vi "VFP.vi"() -> ()   [LabVIEW 2009]
uses:
  states/InitializationStates.ctl
  Instance           6 11Saved   VFP .vi
  Instance          21 11Saved   VFP .vi
  Instance           8 11Saved   VFP .vi
  <vilib>/Utility/error.llb/DialogType.ctl
  states/DataAcqStates.ctl
  Instance           5 11Saved   VFP .vi
  <vilib>/registry/registry.llb/Registry SAM.ctl
  <vilib>/registry/registry.llb/Registry RtKey.ctl
  <vilib>/registry/registry.llb/Read Registry Value Simple STR.vi
  Instance          20 11Saved   VFP .vi
  <vilib>/Utility/error.llb/whitespace.ctl
  <vilib>/Analysis/NI_AALPro.lvlib
panel:
  out "Control Amp Overload":bool caption="CA"
  out "Current Overload":bool caption="I"
  out "Voltage Overload":bool caption="V"
  in  "Select Graph":u16(ring) items=["V Vs. T, I vs. T", "I vs. V", "V vs. I"]
  in  "Log Data To File":bool
  out "Family":string
  out "Vf History":sgl[](array[numeric])
  out "Im History":sgl[](array[numeric])
  out "XY Graph Flipped?":bool
  in  "CA Speed":u16(ring)
  in  "I/E Stability":u16(ring)=2 items=["Fast", "Medium Fast", "Normal", "Slow"]
  in  "IchOffsetEnable":bool
  in  "VchOffsetEnable":bool
  in  "Ich Offset":sgl step=0.1 format="%^.3e"
  in  "Vch Offset":sgl step=0.1 format="%^.3e"
  in  "Ich Filter":u16(ring)
  in  "Vch Filter":u16(ring)
  in  "Ich Autorange":bool
  in  "Vch Autorange":bool
  in  "I/E Autorange":bool
  in  "I/E Range":u16(ring)
  in  "Ich Range":u16(ring)
  in  "Vch Range":u16(ring)
  in  "Device":u16(ring)
  in  "CtrlMode":u32(ring)=1 items=["Galvanostat", "Potentiostat", "ZRA"]
  in  "Continuous":bool=TRUE
  in  "Acq. Frequency":dbl=100.0 caption="Hz" min=0.001667 max=10000.0 step=1.0 format="%.3f"
  in  "Cycles":u32=1 min=1 step=1
  in  "Signal Type":u16(ring) items=["Sine Wave"=0, "Cosine Wave"=1, "Triangle"=2, "Square Wave"=3, "Sawtooth"=4, "Ramp"=5, "Single Point"=7, "From File"=8]
  in  "Filename":path
  in  "Phase Offset":dbl caption="Degrees" step=1.0 format="%.3f"
  in  "DC Offset":dbl caption="V" step=0.1 format="%^.3e"
  in  "Amplitude":dbl=0.1 caption="V" step=0.1 format="%^.3e"
  in  "Signal Frequency":dbl=1.0 caption="Hz" min=5e-05 max=300000.0 step=0.5 format="%.3f"
  in  "Final":dbl=1.0 caption="V" step=0.1 format="%^.3e"
  in  "Initial":dbl caption="V" step=0.1 format="%^.3e"
  in  "Duty Cycle":dbl=50.0 caption="Percent" min=0.0 max=100.0 step=0.1 format="%.3f"
  in  "Scan Rate":dbl=1.0 caption="V/s" step=0.01 format="%_3f"
  in  "Cell State":bool
  in  "Auto Cell Switch":bool=TRUE
  in  "Start/Stop":bool caption="Start"
  out "Confirm Exit?":bool
  out "Vs. T":sgl[][](graph)
  out "I vs. V":cluster{dbl, dbl}[](graph)
  out "SetCell":bool
  out "Cell Val Change NewVal":bool
  out "Version":string
  in  "[user-defined codes]":u32[](array[numeric])=[3758096430]
  in  "[user-defined descriptions]":string[](array[string])=["Device Not Authorized"]
  out "Taking Data":bool
  out "Front Panel Window:Title":string="Gamry Instruments Virtual Front Panel"
  in  "Log File":path
  out "Device Gone":bool
  out "Index of Device (Device Change)":i32
  out "milliseconds to wait":u32=150
  in  "Close":bool
  out "From File Refnum":refnum<file>
  out "Data Handlers":T1
  out "Log File Refnum":refnum<file>
  out "ForcePstatFunctionUpdate":bool
  out "File Data":string
  out "Device List Change Callback":refnum<k27>
  in  "Device List Change":bool
  out "Device Open":bool
  out "Section":string
  in  "GAMRYCOMLib.IGamrySignalArray":refnum<k7>
  in  "GAMRYCOMLib.IGamryDtaqIv":refnum<k7>
  in  "GAMRYCOMLib.IGamryPstat":refnum<k7>
  in  "GAMRYCOMLib.IGamryDeviceList":refnum<k7>
  out "DataDone Callback":refnum<k27>
  out "DataDone?":bool
  out "Dtaq Graph Callback":refnum<k27>
  in  "GAMRYCOMLib.IGamrySignal":refnum<k7>
  out "Signal":refnum<k7>
  out "Dtaq":refnum<k7>
  out "Pstat":refnum<k7>
  out "Device List":refnum<k7>
  out "First I/E Range":i32
  out "Section List":string[](array[string])=["PC5600-00002"]
  # "Overloads"
  # "Data Acquisition"
  # "Signal Generation"
  # "Device Settings"
  # "Experiment Control"
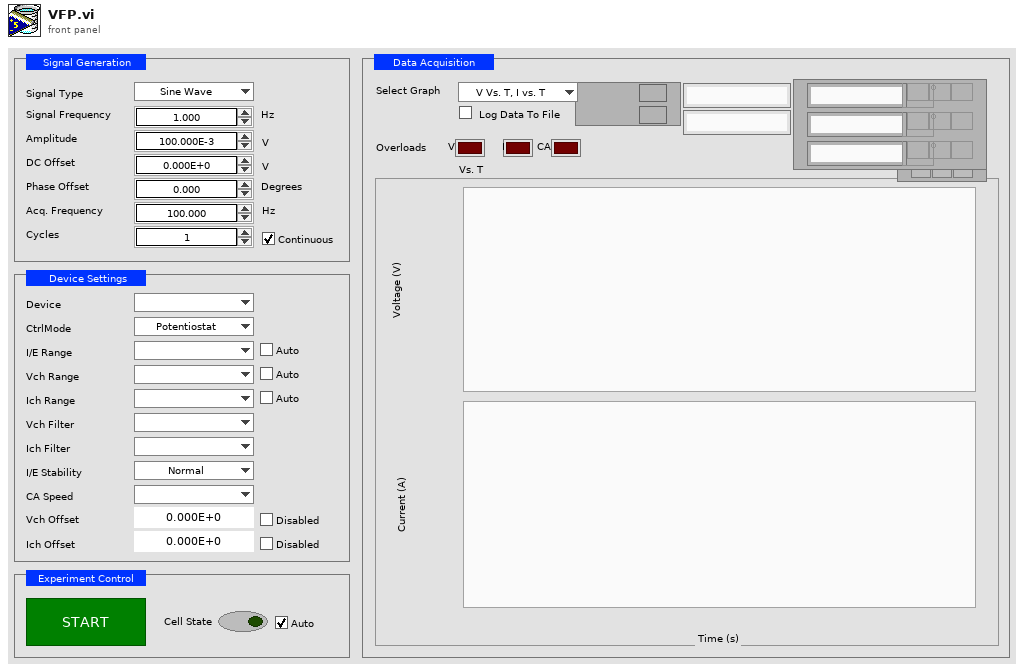
[diagram p1: front panel]
types:
  T1 = cluster{"Vs. T":refnum<vi>, "I vs. V":refnum<vi>, "Log File Refnum":refnum<vi>}
  T2 = typedef "InitializationStates.ctl" = enum16{"Initialize COM", "Load Device List", "Load Range Strings", "Setup Ranges", "Adjust Menu", "STOP"}
  T3 = typedef "DataAcqStates.ctl" = enum16{"Initialize", "Initialize Objects", "Generate Signal", "Data Acq Setup", "Acquire Data", "Cleanup", "STOP"}
  T4 = typedef "Registry SAM.ctl" = enum32{"KEY_QUERY_VALUE", "KEY_SET_VALUE", "KEY_CREATE_SUB_KEY", "KEY_ENUMERATE_SUB_KEYS", "KEY_NOTIFY", "KEY_CREATE_LINK", "KEY_READ", "KEY_WRITE", "KEY_ALL_ACCESS", "KEY_READ | KEY_WRITE"}
  T5 = typedef "Registry RtKey.ctl" = enum32{"HKEY_CLASSES_ROOT", "HKEY_CURRENT_USER", "HKEY_LOCAL_MACHINE", "HKEY_USERS", "HKEY_PERFORMANCE_DATA", "HKEY_CURRENT_CONFIG", "HKEY_DYN_DATA"}
  T6 = enum16{"open", "open or create", "create or replace", "create", "open (read only)"}
  T7 = cluster{"I/E Ranges":string[], "First I/E Range":i32, "VchRanges":string[], "IchRanges":string[], "AchRanges":string[], "VchFilters":string[], "IchFilters":string[], "AchFilters":string[], "Family":string, "CA Speeds":string[]}
  T8 = enum32{"existing file", "new file", "new or existing file", "existing dir", "new dir", "new or existing dir", "existing file (use LLBs)", "new file (use LLBs)", "new or existing file (use LLBs)", "new or existing file or directory (use LLBs)"}
  T9 = typedef "Registry refnum.ctl" = refnum<k1>
  T10 = typedef "whitespace.ctl" = u16
  T11 = cluster{"I Overload":bool, "CA Overload":bool, "V Overload":bool, "I ADC Railed":bool, "V ADC Railed":bool}
  T12 = enum32{"invalid app kind", "Development System", "Run Time System", "Student Edition", "Embedded LabVIEW", "Evaluation", "Custom"}
  T13 = typedef "DialogType.ctl" = u16
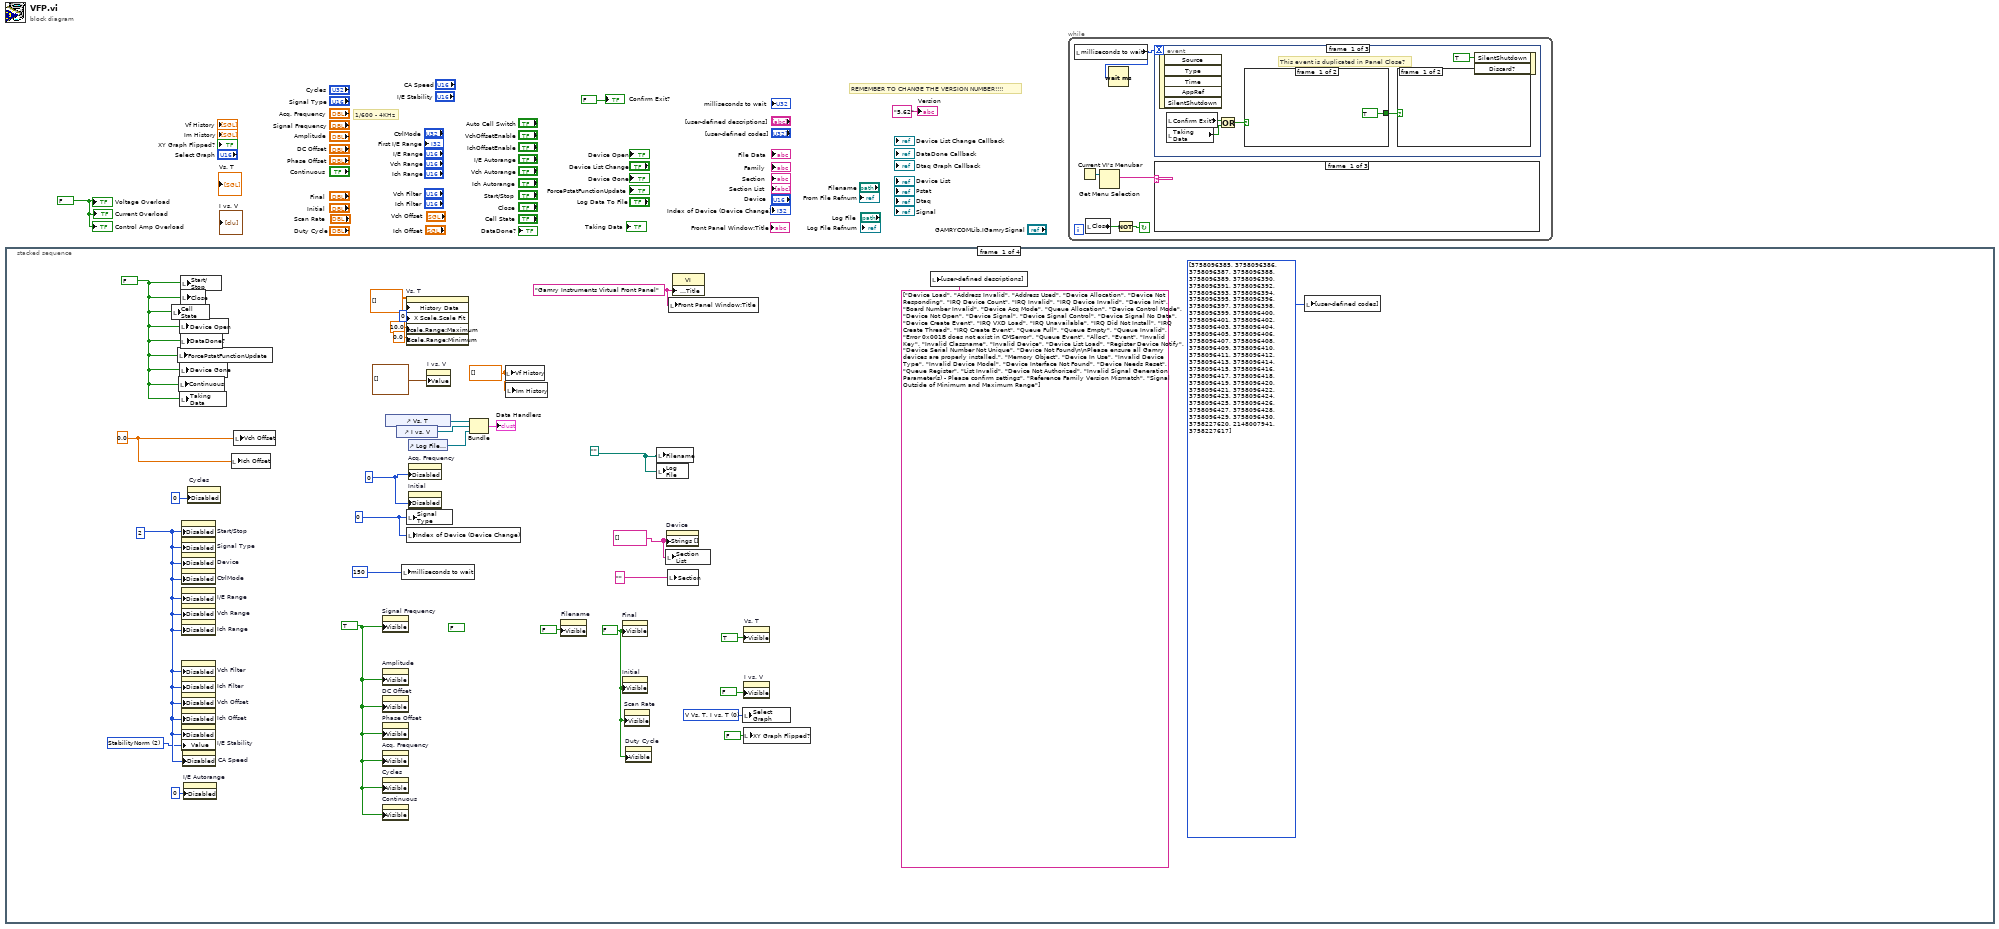
[diagram p0: block diagram]
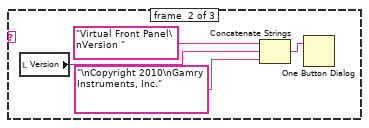
[diagram p2: hidden frame]
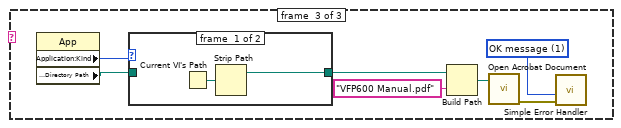
[diagram p3: hidden frame]
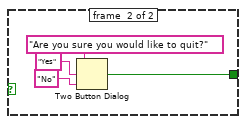
[diagram p5: hidden frame]
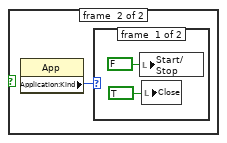
[diagram p6: hidden frame]
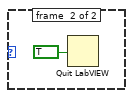
[diagram p7: hidden frame]
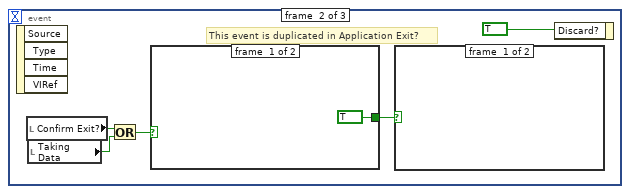
[diagram p8: hidden frame]
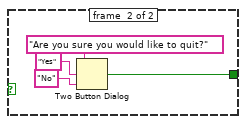
[diagram p9: hidden frame]
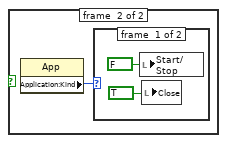
[diagram p10: hidden frame]
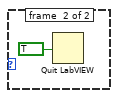
[diagram p11: hidden frame]
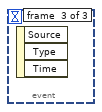
[diagram p12: hidden frame]
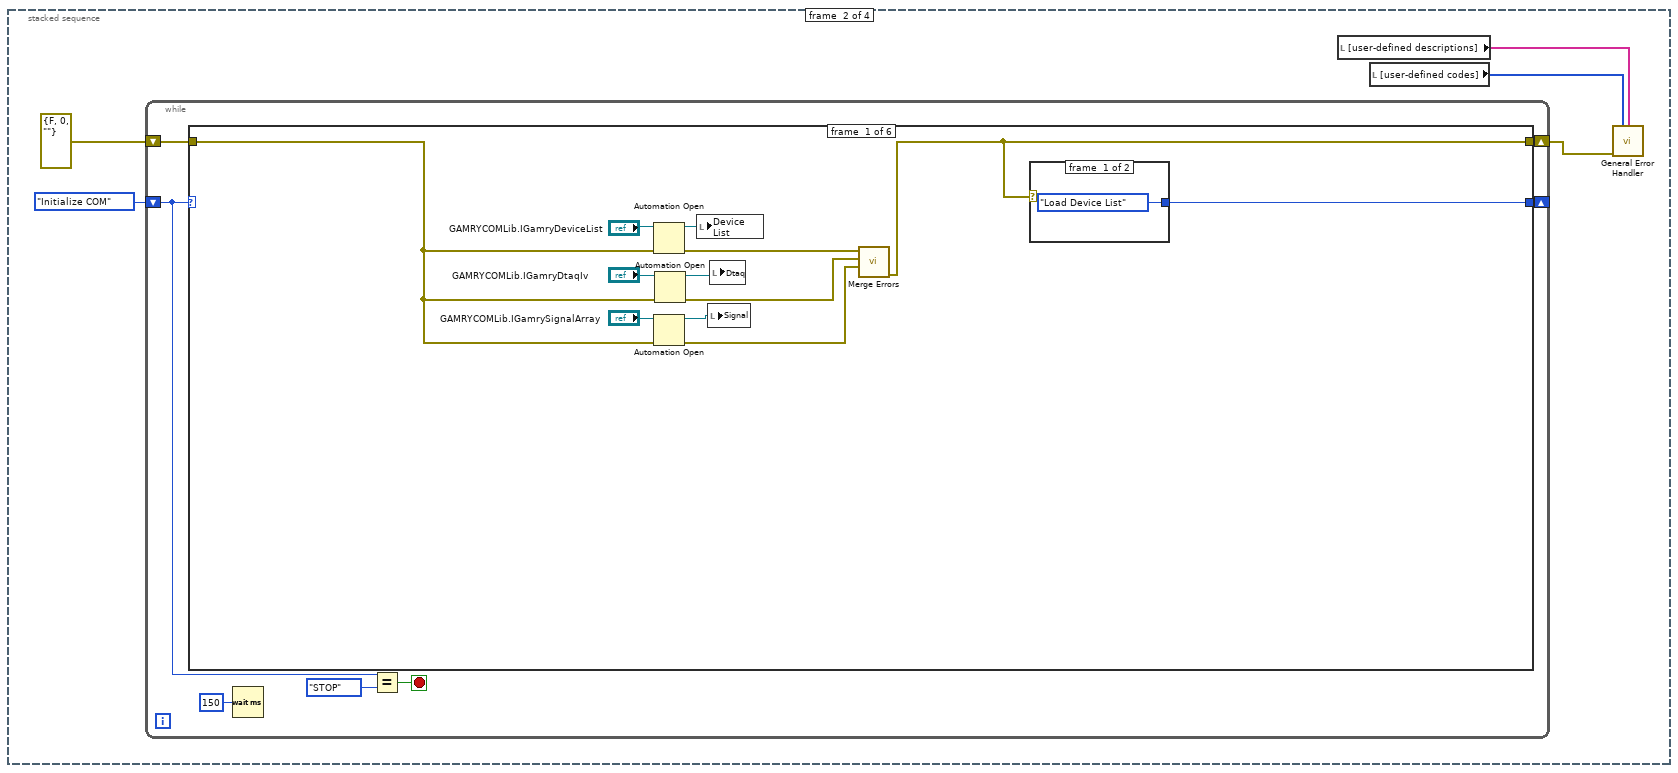
[diagram p13: hidden frame]
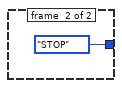
[diagram p14: hidden frame]
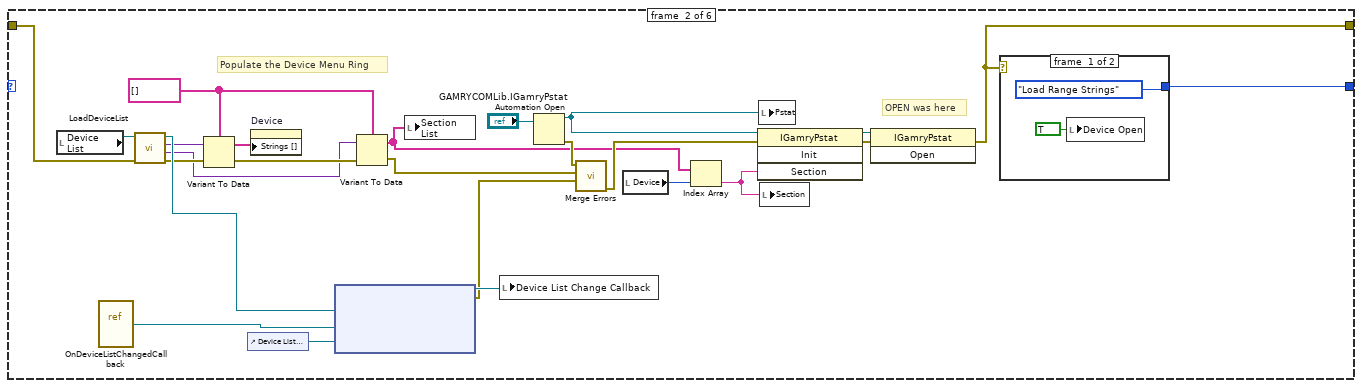
[diagram p15: hidden frame]
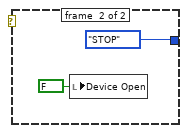
[diagram p16: hidden frame]
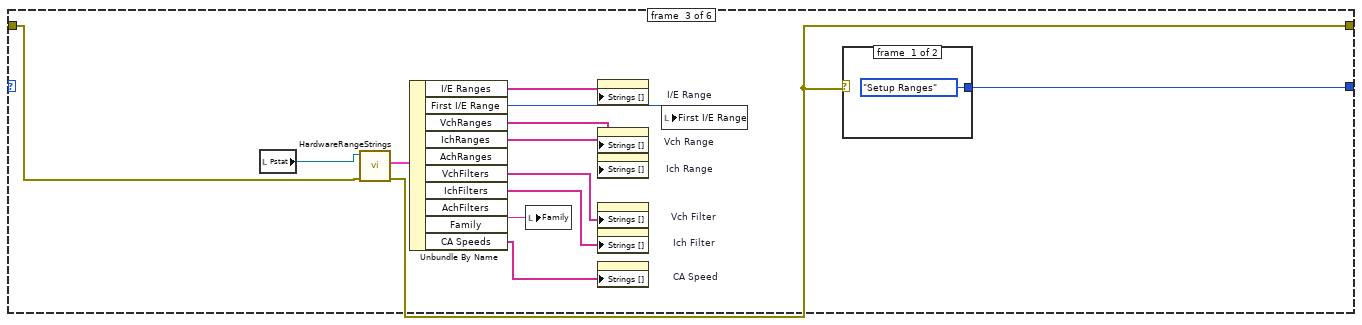
[diagram p17: hidden frame]
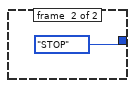
[diagram p18: hidden frame]
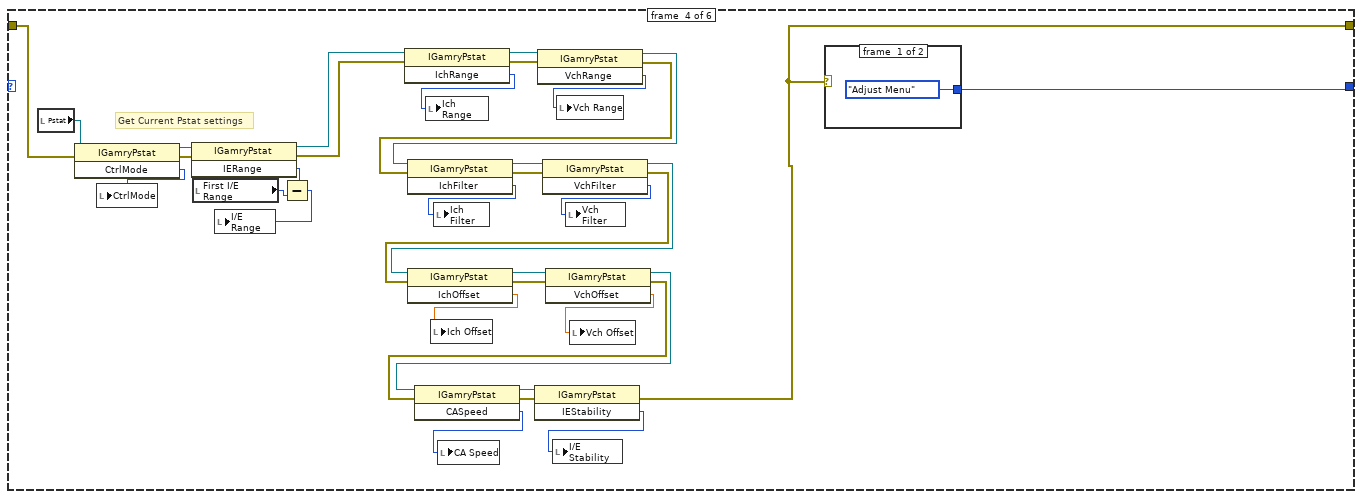
[diagram p19: hidden frame]
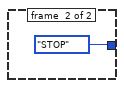
[diagram p20: hidden frame]
diagram:
  w1 = FALSE
  # "REMEMBER TO CHANGE THE VERSION NUMBER!!!!"
  # "1/600 - 4KHz"
  n1 = stacked-sequence {
    frame #0 {
      w5 = sgl[] [] ("Vf History")
      w7 = u16 0 items=["V Vs. T, I vs. T", "I vs. V", "V vs. I"] ("Select Graph")
      w12 = path ""
      w13 = 2 items=["StabilityFast", "StabilityMedFast", "StabilityNorm", "StabilitySlow"] ("Stability")
      w20 = "Gamry Instruments Virtual Front Panel" ("Front Panel Window:Title")
      w15 = FALSE ("Visible")
      w8 = u8 0 ("Disabled")
      w14 = u8 2 ("Disabled")
      (unwired) FALSE ("Visible")
      w30 = TRUE ("Visible")
      w34 = sgl 0.0 ("Vch Offset")
      w19 = FALSE ("I/E Autorange 2")
      w24 = u32 0 ("Zero")
      w25 = string[] [] ("Strings []")
      n2 = local write "Cell State"(w19) -> ()
      n3 = local write "ForcePstatFunctionUpdate"(w19) -> ()
      n4 = local write "Continuous"(w19) -> ()
      n5 = local write "Device Open"(w19) -> ()
      n6 = local write "Device Gone"(w19) -> ()
      n7 = local write "Taking Data"(w19) -> ()
      n8 = local write "DataDone?"(w19) -> ()
      n9 = local write "Start/Stop"(w19) -> ()
      n10 = local write "Close"(w19) -> ()
      n11 = property on="Start/Stop" class="Bool (strict)"("Disabled"=w14) -> ()  [unwired: 2 in, 2 out]
      n12 = property on="Signal Type" class="Ring (strict)"("Disabled"=w14) -> ()  [unwired: 2 in, 2 out]
      n13 = property on="Device" class="Ring (strict)"("Disabled"=w14) -> ()  [unwired: 2 in, 2 out]
      n14 = property on="CtrlMode" class="Ring (strict)"("Disabled"=w14) -> ()  [unwired: 2 in, 2 out]
      n15 = property on="I/E Range" class="Ring (strict)"("Disabled"=w14) -> ()  [unwired: 2 in, 2 out]
      n16 = property on="Vch Range" class="Ring (strict)"("Disabled"=w14) -> ()  [unwired: 2 in, 2 out]
      n17 = property on="Ich Range" class="Ring (strict)"("Disabled"=w14) -> ()  [unwired: 2 in, 2 out]
      n18 = property on="Vch Filter" class="Ring (strict)"("Disabled"=w14) -> ()  [unwired: 2 in, 2 out]
      n19 = property on="Ich Filter" class="Ring (strict)"("Disabled"=w14) -> ()  [unwired: 2 in, 2 out]
      n20 = property on="Vch Offset" class="DigNum (strict)"("Disabled"=w14) -> ()  [unwired: 2 in, 2 out]
      n21 = property on="Ich Offset" class="DigNum (strict)"("Disabled"=w14) -> ()  [unwired: 2 in, 2 out]
      n22 = property on="I/E Stability" class="Ring (strict)"("Disabled"=w14, "Value"=w13) -> ()  [unwired: 2 in, 2 out]
      n23 = property on="CA Speed" class="Ring (strict)"("Disabled"=w14) -> ()  [unwired: 2 in, 2 out]
      n24 = property on="I/E Autorange" class="Boolean (strict)"("Disabled"=u8 0) -> ()  [unwired: 2 in, 2 out]
      n25 = property on="Cycles" class="DigNum (strict)"("Disabled"=0) -> ()  [unwired: 2 in, 2 out]
      n26 = local write "Ich Offset"(w34) -> ()
      n27 = local write "Vch Offset"(w34) -> ()
      n28 = property on="Signal Frequency" class="Digital (strict)"("Visible"=w30) -> ()  [unwired: 2 in, 2 out]
      n29 = property on="Amplitude" class="Digital (strict)"("Visible"=w30) -> ()  [unwired: 2 in, 2 out]
      n30 = property on="DC Offset" class="Digital (strict)"("Visible"=w30) -> ()  [unwired: 2 in, 2 out]
      n31 = property on="Phase Offset" class="Digital (strict)"("Visible"=w30) -> ()  [unwired: 2 in, 2 out]
      n32 = property on="Acq. Frequency" class="Digital (strict)"("Visible"=w30) -> ()  [unwired: 2 in, 2 out]
      n33 = property on="Cycles" class="DigNum (strict)"("Visible"=w30) -> ()  [unwired: 2 in, 2 out]
      n34 = property on="Continuous" class="Boolean (strict)"("Visible"=w30) -> ()  [unwired: 2 in, 2 out]
      n35 = control-ref of="Vs. T"() -> (w33:refnum<vi>)
      n36 = control-ref of="I vs. V"() -> (w32:refnum<vi>)
      n37 = local write "milliseconds to wait"(u32 150 ("milliseconds to wait")) -> ()
      n38 = property on="Vs. T" class="WFChart (strict)"("History Data"=sgl[][] [], "X Scale.Scale Fit"=u8 0, "X Scale.Range:Maximum"=10.0, "X Scale.Range:Minimum"=0.0) -> ()  [unwired: 2 in, 2 out]
      n39 = local write "Index of Device (Device Change)"(w24) -> ()
      n40 = local write "Signal Type"(w24) -> ()
      n41 = control-ref of="Log File Refnum"() -> (w28:refnum<vi>)
      n42 = property on="Acq. Frequency" class="Digital (strict)"("Disabled"=w8) -> ()  [unwired: 2 in, 2 out]
      n43 = property on="Initial" class="DigNum (strict)"("Disabled"=w8) -> ()  [unwired: 2 in, 2 out]
      n44 = property on="I vs. V" class="XYGraph (strict)"("Value"=cluster{dbl, dbl}[] [] ("I vs. V")) -> ()  [unwired: 2 in, 2 out]
      n45 = Bundle("Vs. T"=w33, "I vs. V"=w32, "Log File Refnum"=w28) -> (→"Data Handlers":T1)  [unwired: 1 in]
      n46 = local write "Vf History"(w5) -> ()
      n47 = local write "Im History"(w5) -> ()
      n48 = property on="Filename" class="Path"("Visible"=FALSE) -> ()  [unwired: 2 in, 2 out]
      n49 = property on="Final" class="Digital (strict)"("Visible"=w15) -> ()  [unwired: 2 in, 2 out]
      n50 = property on="Initial" class="Digital (strict)"("Visible"=w15) -> ()  [unwired: 2 in, 2 out]
      n51 = property on="Scan Rate" class="Digital (strict)"("Visible"=w15) -> ()  [unwired: 2 in, 2 out]
      n52 = property on="Duty Cycle" class="DigNum (strict)"("Visible"=w15) -> ()  [unwired: 2 in, 2 out]
      n53 = local write "Filename"(w12) -> ()
      n54 = local write "Log File"(w12) -> ()
      n55 = local write "Section List"(w25) -> ()
      n56 = property on="Device" class="Ring (strict)"("Strings []"=w25) -> ()  [unwired: 2 in, 2 out]
      n57 = local write "Section"("" ("Section")) -> ()
      n58 = local write "Front Panel Window:Title"(w20) -> ()
      n59 = property class="VI"("Front Panel Window:Title"=w20) -> ()  [unwired: 2 in, 2 out]
      n60 = local write "Select Graph"(w7) -> ()
      n61 = local write "XY Graph Flipped?"(FALSE ("XY Graph Flipped?")) -> ()
      n62 = property on="Vs. T" class="WaveformChart (strict)"("Visible"=TRUE) -> ()  [unwired: 2 in, 2 out]
      n63 = property on="I vs. V" class="XYGraph (strict)"("Visible"=FALSE) -> ()  [unwired: 2 in, 2 out]
      n64 = local write "[user-defined descriptions]"(string[] ["Device Load", "Address Invalid", "Address Used", "Device Allocation", "Device Not Responding", "IRQ Device Count", "IRQ Invalid", "IRQ Device Invalid", "Device Init", "Board Number Invalid", "Device Acq Mode", "Queue Allocation", "Device Control Mode", "Device Not Open", "Device Signal", "Device Signal Control", "Device Signal No Data", "Device Create Event", "IRQ VXD Load", "IRQ Unavailable", "IRQ Did Not Install", "IRQ Create Thread", "IRQ Create Event", "Queue Full", "Queue Empty", "Queue Invalid", "Error 0x001B does not exist in CMSerror", "Queue Event", "Alloc", "Event", "Invalid Key", "Invalid Classname", "Invalid Device", "Device List Load", "Register Device Notify", "Device Serial Number Not Unique", "Device Not Found\n\nPlease ensure all Gamry devices are properly installed.", "Memory Object", "Device In Use", "Invalid Device Type", "Invalid Device Model", "Device Interface Not Found", "Device Needs Reset", "Queue Register", "List Invalid", "Device Not Authorized", "Invalid Signal Generation Parameter(s) - Please confirm settings", "Reference Family Version Mismatch", "Signal Outside of Minimum and Maximum Range"] ("[user-defined descriptions]")) -> ()
      n65 = local write "[user-defined codes]"(u32[] [3758096385, 3758096386, 3758096387, 3758096388, 3758096389, 3758096390, 3758096391, 3758096392, 3758096393, 3758096394, 3758096395, 3758096396, 3758096397, 3758096398, 3758096399, 3758096400, 3758096401, 3758096402, 3758096403, 3758096404, 3758096405, 3758096406, 3758096407, 3758096408, 3758096409, 3758096410, 3758096411, 3758096412, 3758096413, 3758096414, 3758096415, 3758096416, 3758096417, 3758096418, 3758096419, 3758096420, 3758096421, 3758096422, 3758096423, 3758096424, 3758096425, 3758096426, 3758096427, 3758096428, 3758096429, 3758096430, 3758227620, 2148007941, 3758227617] ("[user-defined codes]")) -> ()
    }
    frame #1 {
      n66 = while {
        shift-right: [w41] -> _
        shift-left: InitializationStates."Initialize COM" ("Initialization States") -> [w47]
        shift-right: [w43] -> w36
        shift-left: errorcluster {"status"=FALSE, "code"=0, "source"=""} ("error out") -> [w42]
        stop <- w45 stop-if-true
        n67 = case shown="\"Adjust Menu\"" w47 {
          tunnel: [w49 w62 w91 w106 w142 w161] -> w43
          tunnel: w42 -> [w50 w67 w93 w133 w143 w161]
          tunnel: [w48 w65 w97 w132 w151 InitializationStates."STOP" ("Initialization States")] -> w41
          frame #0 {
            n68 = Automation Open(error in (no error)=w50, Automation Refnum="GAMRYCOMLib.IGamryDeviceList") -> (Automation Refnum=w59:refnum<k7>, error out=w56:errorcluster)  [unwired: 2 in]
            n69 = Automation Open(error in (no error)=w50, Automation Refnum="GAMRYCOMLib.IGamrySignalArray") -> (Automation Refnum=w52:refnum<k7>, error out=w58:errorcluster)  [unwired: 2 in]
            n70 = Automation Open(error in (no error)=w50, Automation Refnum="GAMRYCOMLib.IGamryDtaqIv") -> (Automation Refnum=w51:refnum<k7>, error out=w57:errorcluster)  [unwired: 2 in]
            n71 = local write "Device List"(w59) -> ()
            n72 = local write "Signal"(w52) -> ()
            n73 = local write "Dtaq"(w51) -> ()
            n74 = call <vilib>:"Merge Errors.vi"("error in 3 (no error)"=w58, "error in 2 (no error)"=w57, "error in 1 (no error)"=w56) -> ("error out"=w49:errorcluster)  [unwired: 4 in]
            n75 = case shown="No Error" w49 {
              tunnel: [InitializationStates."Load Device List" ("Initialization States") InitializationStates."STOP" ("Initialization States")] -> w48
              frame #0 {
              }
              frame #1 {
              }
            }
          }
          frame #1 {
            w69 = string[] []
            # "OPEN was here"
            # "Populate the Device Menu Ring"
            n76 = local read "Device List"() -> (w86:refnum<k7>)
            n77 = vi-ref "OnDeviceListChangedCallback.vi"() -> ("vi reference"=w75:refnum<vi>)
            n78 = call "LoadDeviceList.vi"("Error In"=w67, "GAMRYCOMLib.IGamryDeviceList In"=w86) -> ("Error Out"=w82:errorcluster, "EnumSections"=w81:variant, "EnumLabels"=w80:variant, "GAMRYCOMLib.IGamryDeviceList Out"=w85:refnum<k7>)  [unwired: 4 in]
            n79 = Variant To Data(error in=w82, Variant=w80, type=w69) -> (error out=w84:errorcluster, data=w68:string[])
            n80 = control-ref of="Device List Change"() -> (w74:refnum<vi>)
            n81 = property on="Device" class="Ring (strict)"("Strings []"=w68) -> ()  [unwired: 2 in, 2 out]
            n82 = node(w85, w75, w74) -> (w76:refnum<k27>, w66:errorcluster)  [unwired: 2 in]
            n83 = Variant To Data(error in=w84, Variant=w81, type=w69) -> (error out=w83:errorcluster, data=w77:string[])
            n84 = local write "Section List"(w77) -> ()
            n85 = local write "Device List Change Callback"(w76) -> ()
            n86 = Automation Open(Automation Refnum="GAMRYCOMLib.IGamryPstat") -> (Automation Refnum=w73:refnum<k7>, error out=w78:errorcluster)  [unwired: 3 in]
            n87 = call <vilib>:"Merge Errors.vi"("error in 3 (no error)"=w66, "error in 2 (no error)"=w83, "error in 1 (no error)"=w78) -> ("error out"=w79:errorcluster)  [unwired: 4 in]
            n88 = local read "Device"() -> (w71:u16)
            n89 = Index Array(array=w77, index=w71) -> (element=w72:string)
            n90 = invoke class="IGamryPstat" method="Init"(reference=w73, error in=w79, "Section"=w72) -> (reference out=w63:refnum<k7>, error out=w64:errorcluster)  [unwired: 1 in, 2 out]
            n91 = local write "Pstat"(w73) -> ()
            n92 = local write "Section"(w72) -> ()
            n93 = invoke class="IGamryPstat" method="Open"(reference=w63, error in=w64) -> (error out=w62:errorcluster)  [unwired: 1 in, 2 out]
            n94 = case shown="Error" w62 {
              tunnel: [InitializationStates."Load Range Strings" ("Initialization States") InitializationStates."STOP" ("Initialization States")] -> w65
              frame #0 {
                n95 = local write "Device Open"(TRUE ("Device Open")) -> ()
              }
              frame #1 {
                n96 = local write "Device Open"(FALSE ("Device Open")) -> ()
              }
            }
          }
          frame #2 {
            n97 = local read "Pstat"() -> (w94:refnum<k7>)
            n98 = call "HardwareRangeStrings.vi"("error in (no error)"=w93, "Pstat IN"=w94) -> ("error out"=w91:errorcluster, "Hardware Strings"=w92:T7)  [unwired: 7 in, 1 out]
            n99 = Unbundle By Name(w92) -> ("I/E Ranges"=w101:string[], "First I/E Range"=w98:i32, "VchRanges"=w99:string[], "IchRanges"=w100:string[], "VchFilters"=w102:string[], "IchFilters"=w103:string[], "Family"=w95:string, "CA Speeds"=w96:string[])  [unwired: 2 out]
            n100 = local write "Family"(w95) -> ()
            n101 = property on="I/E Range" class="Ring (strict)"("Strings []"=w101) -> ()  [unwired: 2 in, 2 out]
            n102 = property on="Vch Range" class="Ring (strict)"("Strings []"=w99) -> ()  [unwired: 2 in, 2 out]
            n103 = property on="Ich Range" class="Ring (strict)"("Strings []"=w100) -> ()  [unwired: 2 in, 2 out]
            n104 = property on="Vch Filter" class="Ring (strict)"("Strings []"=w102) -> ()  [unwired: 2 in, 2 out]
            n105 = property on="Ich Filter" class="Ring (strict)"("Strings []"=w103) -> ()  [unwired: 2 in, 2 out]
            n106 = property on="CA Speed" class="Ring (strict)"("Strings []"=w96) -> ()  [unwired: 2 in, 2 out]
            n107 = local write "First I/E Range"(w98) -> ()
            n108 = case shown="No Error" w91 {
              tunnel: [InitializationStates."Setup Ranges" ("Initialization States") InitializationStates."STOP" ("Initialization States")] -> w97
              frame #0 {
              }
              frame #1 {
              }
            }
          }
          frame #3 {
            # "Get Current Pstat settings"
            n109 = local read "Pstat"() -> (w134:refnum<k7>)
            n110 = invoke class="IGamryPstat" method="CtrlMode"(reference=w134, error in=w133) -> (reference out=w138:refnum<k7>, error out=w139:errorcluster, "CtrlMode"=w136:i32)  [unwired: 1 in]
            n111 = local write "CtrlMode"(w136) -> ()
            n112 = invoke class="IGamryPstat" method="IERange"(reference=w138, error in=w139) -> (reference out=w108:refnum<k7>, error out=w107:errorcluster, "IERange"=w135:i32)  [unwired: 1 in]
            n113 = local read "First I/E Range"() -> (w131:i32)
            n114 = Subtract(x=w135, y=w131) -> (x-y=w137:i32)
            n115 = local write "I/E Range"(w137) -> ()
            n116 = invoke class="IGamryPstat" method="IchRange"(reference=w108, error in=w107) -> (reference out=w113:refnum<k7>, error out=w112:errorcluster, "IchRange"=w110:i32)  [unwired: 1 in]
            n117 = local write "Ich Range"(w110) -> ()
            n118 = invoke class="IGamryPstat" method="VchRange"(reference=w113, error in=w112) -> (reference out=w126:refnum<k7>, error out=w109:errorcluster, "VchRange"=w111:i32)  [unwired: 1 in]
            n119 = invoke class="IGamryPstat" method="IchFilter"(reference=w126, error in=w109) -> (reference out=w121:refnum<k7>, error out=w120:errorcluster, "IchFilter"=w122:i32)  [unwired: 1 in]
            n120 = local write "Ich Filter"(w122) -> ()
            n121 = invoke class="IGamryPstat" method="VchFilter"(reference=w121, error in=w120) -> (reference out=w128:refnum<k7>, error out=w127:errorcluster, "VchFilter"=w123:i32)  [unwired: 1 in]
            n122 = invoke class="IGamryPstat" method="IchOffset"(reference=w128, error in=w127) -> (reference out=w118:refnum<k7>, error out=w119:errorcluster, "IchOffset"=w124:sgl)  [unwired: 1 in]
            n123 = local write "Ich Offset"(w124) -> ()
            n124 = invoke class="IGamryPstat" method="VchOffset"(reference=w118, error in=w119) -> (reference out=w130:refnum<k7>, error out=w129:errorcluster, "VchOffset"=w125:sgl)  [unwired: 1 in]
            n125 = invoke class="IGamryPstat" method="CASpeed"(reference=w130, error in=w129) -> (reference out=w114:refnum<k7>, error out=w115:errorcluster, "CASpeed"=w117:i32)  [unwired: 1 in]
            n126 = local write "CA Speed"(w117) -> ()
            n127 = invoke class="IGamryPstat" method="IEStability"(reference=w114, error in=w115) -> (error out=w106:errorcluster, "IEStability"=w116:i32)  [unwired: 1 in, 1 out]
            n128 = local write "I/E Stability"(w116) -> ()
            n129 = local write "Vch Range"(w111) -> ()
            n130 = local write "Vch Filter"(w123) -> ()
            n131 = local write "Vch Offset"(w125) -> ()
            n132 = case shown="No Error" w106 {
              tunnel: [InitializationStates."Adjust Menu" ("Initialization States") InitializationStates."STOP" ("Initialization States")] -> w132
              frame #0 {
              }
              frame #1 {
              }
            }
          }
          frame #4 {
            n133 = local read "CtrlMode"() -> (w150:u32)
            n134 = case shown="1, Default" w150 {
              tunnel: ["V" ("Caption.Text") "A" ("Caption.Text")] -> w149
              tunnel: ["V/s" ("Caption.Text") "A/s" ("Caption.Text")] -> w148
              frame #0 {
              }
              frame #1 {
              }
            }
            n135 = property on="Amplitude" class="Digital (strict)"(error in=w143, "Caption.Text"=w149) -> (error out=w147:errorcluster)  [unwired: 1 in, 1 out]
            n136 = property on="DC Offset" class="Digital (strict)"(error in=w147, "Caption.Text"=w149) -> (error out=w146:errorcluster)  [unwired: 1 in, 1 out]
            n137 = property on="Initial" class="DigNum (strict)"(error in=w146, "Caption.Text"=w149) -> (error out=w145:errorcluster)  [unwired: 1 in, 1 out]
            n138 = property on="Final" class="Digital (strict)"(error in=w145, "Caption.Text"=w149) -> (error out=w144:errorcluster)  [unwired: 1 in, 1 out]
            n139 = property on="Scan Rate" class="Digital (strict)"(error in=w144, "Caption.Text"=w148) -> (error out=w142:errorcluster)  [unwired: 1 in, 1 out]
            n140 = case shown="Error" w142 {
              tunnel: [InitializationStates."STOP" ("Initialization States") InitializationStates."STOP" ("Initialization States")] -> w151
              frame #0 {
                w156 = u8 0 ("Disabled")
                # "Enable appropriate menu stuff"
                n141 = property on="Start/Stop" class="Bool (strict)"("Disabled"=w156) -> ()  [unwired: 2 in, 2 out]
                n142 = property on="Device" class="Ring (strict)"("Disabled"=w156) -> ()  [unwired: 2 in, 2 out]
                n143 = property on="CtrlMode" class="Ring (strict)"("Disabled"=w156) -> ()  [unwired: 2 in, 2 out]
                n144 = property on="Signal Type" class="Ring (strict)"("Disabled"=w156) -> ()  [unwired: 2 in, 2 out]
                n145 = property on="I/E Range" class="Ring (strict)"("Disabled"=w156) -> ()  [unwired: 2 in, 2 out]
                n146 = property on="Vch Range" class="Ring (strict)"("Disabled"=w156) -> ()  [unwired: 2 in, 2 out]
                n147 = property on="Ich Range" class="Ring (strict)"("Disabled"=w156) -> ()  [unwired: 2 in, 2 out]
                n148 = property on="Vch Filter" class="Ring (strict)"("Disabled"=w156) -> ()  [unwired: 2 in, 2 out]
                n149 = property on="Ich Filter" class="Ring (strict)"("Disabled"=w156) -> ()  [unwired: 2 in, 2 out]
                n150 = property on="Vch Offset" class="DigNum (strict)"("Disabled"=w156) -> ()  [unwired: 2 in, 2 out]
                n151 = property on="Ich Offset" class="DigNum (strict)"("Disabled"=w156) -> ()  [unwired: 2 in, 2 out]
                n152 = property on="I/E Stability" class="Ring (strict)"("Disabled"=w156) -> ()  [unwired: 2 in, 2 out]
                n153 = property on="CA Speed" class="Ring (strict)"("Disabled"=w156) -> ()  [unwired: 2 in, 2 out]
              }
              frame #1 {
                w160 = u16 0 items=[""] ("Device")
                w158 = u8 2 ("Disabled")
                # "Disable appropriate menu stuff"
                n154 = property on="Start/Stop" class="Bool (strict)"("Disabled"=w158) -> ()  [unwired: 2 in, 2 out]
                n155 = property on="CtrlMode" class="Ring (strict)"("Disabled"=w158) -> ()  [unwired: 2 in, 2 out]
                n156 = property on="Device" class="Ring (strict)"("Disabled"=w158, "Value"=w160) -> ()  [unwired: 2 in, 2 out]
                n157 = property on="I/E Range" class="Ring (strict)"("Disabled"=w158, "Value"=w160) -> ()  [unwired: 2 in, 2 out]
                n158 = property on="Vch Range" class="Ring (strict)"("Disabled"=w158, "Value"=w160) -> ()  [unwired: 2 in, 2 out]
                n159 = property on="Ich Range" class="Ring (strict)"("Disabled"=w158, "Value"=w160) -> ()  [unwired: 2 in, 2 out]
                n160 = property on="Vch Filter" class="Ring (strict)"("Disabled"=w158, "Value"=w160) -> ()  [unwired: 2 in, 2 out]
                n161 = property on="Ich Filter" class="Ring (strict)"("Disabled"=w158, "Value"=w160) -> ()  [unwired: 2 in, 2 out]
                n162 = property on="Vch Offset" class="DigNum (strict)"("Disabled"=w158) -> ()  [unwired: 2 in, 2 out]
                n163 = property on="Ich Offset" class="DigNum (strict)"("Disabled"=w158) -> ()  [unwired: 2 in, 2 out]
                n164 = property on="I/E Stability" class="Ring (strict)"("Disabled"=w158) -> ()  [unwired: 2 in, 2 out]
                n165 = property on="CA Speed" class="Ring (strict)"("Disabled"=w158) -> ()  [unwired: 2 in, 2 out]
              }
            }
          }
          frame #5 {
          }
        }
        n166 = Wait (ms)(milliseconds to wait=u32 150) -> ()  [unwired: 1 out]
        n167 = Equal?(x=w47, y=InitializationStates."STOP" ("Initialization States")) -> (x = y?=w45:bool)
      }
      n168 = local read "[user-defined descriptions]"() -> (w40:string[])
      n169 = local read "[user-defined codes]"() -> (w39:u32[])
      n170 = call <vilib>:"General Error Handler.vi"("[user-defined codes]"=w39, "[user-defined descriptions]"=w40, "error in (no error)"=w36) -> ()  [unwired: 8 in, 5 out]
    }
    frame #2 {
      n171 = while {
        stop <- w655 continue-if-true
        n172 = local read "milliseconds to wait"() -> (w654:u32)
        n173 = event shown="[0] \"Start/Stop\": Value Change" {
          selector: _ -> [_ _]
          dyn-events: _ -> [_ _]
          timeout: w654 -> [_ _]
          event #0 {
            n174 = event-data() -> ("NewVal"=w657:bool)  [unwired: 1 in, 4 out]
            n175 = case shown="True" w657 {
              frame #0 {
              }
              frame #1 {
                n176 = while {
                  shift-right: [w662] -> _
                  shift-left: DataAcqStates."Initialize" ("Data Acq States") -> [w665]
                  shift-right: [w660] -> _
                  shift-left: errorcluster {"status"=FALSE, "code"=0, "source"=""} ("error in (no error)") -> [w661]
                  stop <- w666 stop-if-true
                  n177 = case shown="\"Generate Signal\"" w665 {
                    tunnel: [DataAcqStates."Initialize Objects" ("Data Acq States") w732 w747 w916 w932 w1019 DataAcqStates."STOP" ("Data Acq States")] -> w662
                    tunnel: w661 -> [w671 w712 w748 w917 w933 w1021 w1057]
                    tunnel: [w671 w722 w746 w914 w931 w1018 w1048] -> w660
                    frame #0 {
                      w668 = path "" ("Log File")
                      w669 = sgl[] [] ("Vf History")
                      w670 = u8 2 ("Disabled")
                      w667 = FALSE
                      # "Initalize Chart and Lists"
                      # "Disable appropriate menu items"
                      n178 = local read "Continuous"() -> (w677:bool)
                      n179 = property on="CtrlMode" class="Ring (strict)"("Disabled"=w670) -> ()  [unwired: 2 in, 2 out]
                      n180 = property on="Log Data To File" class="Boolean (strict)"("Disabled"=w670) -> ()  [unwired: 2 in, 2 out]
                      n181 = property on="Device" class="Ring (strict)"("Disabled"=w670) -> ()  [unwired: 2 in, 2 out]
                      n182 = property on="Acq. Frequency" class="DigNum (strict)"("Disabled"=w670) -> ()  [unwired: 2 in, 2 out]
                      n183 = Select(t=2, s=w677, f=0) -> (s? t:f=w676:i32)
                      n184 = property on="Log File" class="Path"("Value"=w668) -> ()  [unwired: 2 in, 2 out]
                      n185 = property on="Cycles" class="DigNum (strict)"("Disabled"=w676) -> ()  [unwired: 2 in, 2 out]
                      n186 = local read "Log Data To File"() -> (w673:bool)
                      n187 = case shown="True" w673 {
                        tunnel: [FALSE w708] -> w672
                        tunnel: w668 -> [_ _]
                        frame #0 {
                          n188 = local read "Front Panel Window:Title"() -> (w682:string)
                          n189 = property class="VI"("Front Panel Window:Title"=w682) -> ()  [unwired: 2 in, 2 out]
                        }
                        frame #1 {
                          (unwired) T8."new or existing file" ("select mode (2)")
                          n190 = call <vilib>:"Open Registry Key.vi"("security access mask (KEY_READ | KEY_WRITE)"=Registry_SAM."KEY_READ", "subkey"="SOFTWARE\\Microsoft\\Windows\\CurrentVersion\\Explorer\\Shell Folders\\", "root key (HKEY_LOCAL_MACHINE)"=Registry_RtKey."HKEY_LOCAL_MACHINE") -> ("error out"=w689:errorcluster, "refnum out"=w691:T9)  [unwired: 7 in]
                          n191 = call-poly <vilib>:"Read Registry Value Simple.vi"("error in (no error)"=w689, "default data"="C:\\Documents and Settings\\All Users\\Documents\\", "value"="Common Documents", "refnum"=w691) -> ("error out"=w690:errorcluster, "String/Binary data"=w697:string, "refnum out"=w692:T9)  [unwired: 2 in, 1 out]
                          n192 = call <vilib>:"Close Registry Key.vi"("error in (no error)"=w690, "refnum"=w692) -> ()  [unwired: 5 in, 1 out]
                          n193 = Concatenate Strings(w697, "\\My Gamry Data\\" ("string")) -> (w699:string)
                          n194 = local read "Front Panel Window:Title"() -> (w704:string)
                          n195 = String To Path(string=w699) -> (path=w687:path)
                          n196 = File Dialog(6:"*.txt" ("pattern"), 7:"Data File Location" ("prompt"), 9:"logfile.txt" ("default name"), 11:w687) -> (0:w684:errorcluster, 3:w685:path)  [unwired: 3 in, 2 out]
                          n197 = Unbundle(w684) -> ()  [unwired: 3 out]
                          n198 = call <vilib>:"Open_Create_Replace File.vi"("function (open:0)"=T6."create or replace", "file path"=w685) -> ("error out"=w709:errorcluster, "refnum"=w711:refnum<file>)  [unwired: 6 in, 2 out]
                          n199 = Path To String(path=w685) -> (string=w702:string)
                          n200 = local write "Log File Refnum"(w711) -> ()
                          n201 = Concatenate Strings(w704, " - " ("string"), w702) -> (w705:string)
                          n202 = Unbundle By Name(w709) -> ("status"=w706:bool)
                          n203 = local write "Log File"(w685) -> ()
                          n204 = property class="VI"("Front Panel Window:Title"=w705) -> ()  [unwired: 2 in, 2 out]
                          n205 = Empty String/Path?(string/path=w685) -> (empty?=w707:bool)
                          n206 = Or(x=w707, y=w706) -> (x .or. y?=w708:bool)
                        }
                      }
                      n207 = property on="Vs. T" class="WFChart (strict)"("History Data"=sgl[][] []) -> ()  [unwired: 2 in, 2 out]
                      n208 = property on="I vs. V" class="XYGraph (strict)"("Value"=cluster{dbl, dbl}[] [] ("I vs. V")) -> ()  [unwired: 2 in, 2 out]
                      n209 = local write "Vf History"(w669) -> ()
                      n210 = local write "Im History"(w669) -> ()
                      n211 = local write "Control Amp Overload"(w667) -> ()
                      n212 = local write "Voltage Overload"(w667) -> ()
                      n213 = local write "Current Overload"(w667) -> ()
                      n214 = case shown="True" w672 {
                        frame #0 {
                        }
                        frame #1 {
                          n215 = local write "Log Data To File"(FALSE) -> ()
                        }
                      }
                      n216 = call "Log File Error"("Enable"=w672) -> ()  [unwired: 9 in, 2 out]
                    }
                    frame #1 {
                      # "Register a sub VI to handle our DataAvailable and DataDone events"
                      n217 = local read "Pstat"() -> (w713:refnum<k7>)
                      n218 = invoke class="IGamryPstat" method="ModelNo"(reference=w713, error in=w712) -> (reference out=w714:refnum<k7>, error out=w715:errorcluster, "ModelNo"=w718:i32)  [unwired: 1 in]
                      n219 = Equal?(x=w718, y=4) -> (x = y?=w716:bool)
                      n220 = case shown="True" w716 {
                        tunnel: w714 -> [w734 w739]
                        tunnel: w715 -> [w733 w738]
                        tunnel: [w734 w737] -> w720
                        tunnel: [w733 w736] -> w719
                        frame #0 {
                        }
                        frame #1 {
                          n221 = invoke class="IGamryPstat" method="SetExtSrceEnable"(reference=w739, error in=w738, "ExtSrceEnable"=TRUE) -> (reference out=w737:refnum<k7>, error out=w736:errorcluster)  [unwired: 1 in, 2 out]
                        }
                      }
                      n222 = local read "CtrlMode"() -> (w725:u32)
                      n223 = invoke class="IGamryPstat" method="SetCtrlMode"(reference=w720, error in=w719, "CtrlMode"=w725) -> (reference out=w727:refnum<k7>, error out=w726:errorcluster, "SetCtrlMode"=w723:i32)  [unwired: 1 in, 1 out]
                      n224 = local write "CtrlMode"(w723) -> ()
                      n225 = local read "Dtaq"() -> (w724:refnum<k7>)
                      n226 = invoke class="IGamryDtaqIv" method="Init"(reference=w724, error in=w726, "Pstat"=w727) -> (reference out=w731:refnum<k7>, error out=w730:errorcluster)  [unwired: 1 in, 2 out]
                      n227 = control-ref of="DataDone?"() -> (w728:refnum<vi>)
                      n228 = vi-ref "DtaqDataDoneCallback - DtaqIV.vi"() -> ("vi reference"=w721:refnum<vi>)
                      n229 = node(w730, w731, w721, w728) -> (w729:refnum<k27>, w722:errorcluster)  [unwired: 1 in]
                      n230 = local write "DataDone Callback"(w729) -> ()
                      n231 = case shown="No Error" w722 {
                        tunnel: [DataAcqStates."Generate Signal" ("Data Acq States") DataAcqStates."STOP" ("Data Acq States")] -> w732
                        frame #0 {
                        }
                        frame #1 {
                        }
                      }
                    }
                    frame #2 {
                      # "Nyquist Criterion"
                      n232 = local read "Signal Frequency"() -> (w744:dbl)
                      n233 = local read "Acq. Frequency"() -> (w745:dbl)
                      n234 = local read "Signal Type"() -> (w742:u16)
                      n235 = case shown="0, 1, 3, 4" w742 {
                        tunnel: w745 -> [_ w754]
                        tunnel: w744 -> [_ w752]
                        tunnel: [TRUE w750] -> w743
                        frame #0 {
                        }
                        frame #1 {
                          n236 = Multiply(x=2.0, y=w752) -> (x*y=w753:dbl)
                          n237 = Greater?(x=w754, y=w753) -> (0:w750:bool)
                        }
                      }
                      n238 = case shown="True" w743 {
                        tunnel: w744 -> [_ w778]
                        tunnel: w745 -> [_ w762]
                        tunnel: w748 -> [w756 w770]
                        tunnel: [DataAcqStates."STOP" ("Data Acq States") w768] -> w747
                        tunnel: [w755 w759] -> w746
                        frame #0 {
                          n239 = call "Nyquist Criterion"("error in (no error)"=w756, "Enable"=TRUE) -> ("error out"=w755:errorcluster)  [unwired: 8 in, 1 out]
                        }
                        frame #1 {
                          n240 = local read "Amplitude"() -> (w779:dbl)
                          n241 = local read "Continuous"() -> (w776:bool)
                          n242 = local read "Signal Type"() -> (w775:u16)
                          n243 = local read "Cycles"() -> (w777:u32)
                          n244 = local read "Phase Offset"() -> (w781:dbl)
                          n245 = local read "Duty Cycle"() -> (w792:dbl)
                          n246 = local read "DC Offset"() -> (w780:dbl)
                          n247 = local read "Scan Rate"() -> (w782:dbl)
                          n248 = local read "Final"() -> (w783:dbl)
                          n249 = local read "Initial"() -> (w784:dbl)
                          n250 = case shown="8" w775 {
                            selector: w775 -> [w817 w823 w857 w866 _ _ _]
                            tunnel: w776 -> [w819 w833 w859 _ _ w894 w908]
                            tunnel: w777 -> [w818 w832 w858 _ _ w893 w907]
                            tunnel: w762 -> [w808 w831 w856 w863 w882 w892 w913]
                            tunnel: w778 -> [w807 _ w847 _ _ _ _]
                            tunnel: w779 -> [w816 _ w855 _ _ _ _]
                            tunnel: w780 -> [w815 _ w854 _ w877 _ _]
                            tunnel: w781 -> [w814 _ w853 _ _ _ _]
                            tunnel: w782 -> [_ w830 _ w872 _ _ _]
                            tunnel: w783 -> [_ w829 _ w871 _ _ _]
                            tunnel: w784 -> [_ w828 _ w870 _ _ _]
                            tunnel: [w813 w826 w852 w868 w880 w889 dbl[] []] -> w785
                            tunnel: [w812 w827 w851 1 ("t") -1 ("t") w890 w906] -> w795
                            tunnel: [w811 w825 w850 w864 w879 w891 w912] -> w764
                            tunnel: [w810 w824 w849 w867 0 ("error") 0 ("error") 0 ("error")] -> w791
                            tunnel: w792 -> [_ _ w848 _ _ _ _]
                            frame #0 {
                              # "Sine, Cosine, Sawtooth"
                              n251 = Select(t=-1, s=w819, f=w818) -> (s? t:f=w812:u32)
                              n252 = Reciprocal(x=w807) -> (1/x=w806:dbl)
                              n253 = Reciprocal(x=w808) -> (1/x=w811:dbl)
                              n254 = Multiply(x=w808, y=w806) -> (x*y=w809:dbl)
                              n255 = call <vilib>:"Signal Generator by Duration.vi"("signal type"=w817, "duration"=w806, "# of samples"=w809, "frequency"=w807, "amplitude"=w816, "dc offset"=w815, "phase in"=w814) -> ("signal"=w813:dbl[], "error"=w810:i32)  [unwired: 5 in, 2 out]
                            }
                            frame #1 {
                              # "Triangle"
                              n256 = Select(t=-1, s=w833, f=w832) -> (s? t:f=w827:u32)
                              n257 = Subtract(x=w829, y=w828) -> (x-y=w838:dbl)
                              n258 = Add(x=w829, y=w828) -> (x+y=w834:dbl)
                              n259 = Divide(x=w838, y=w830) -> (x/y=w843:dbl)
                              n260 = Divide(x=w838, y=2.0) -> (x/y=w837:dbl)
                              n261 = Divide(x=w834, y=2.0) -> (x/y=w836:dbl)
                              n262 = Reciprocal(x=w831) -> (1/x=w825:dbl)
                              n263 = Absolute Value(x=w843) -> (abs(x)=w842:dbl)
                              n264 = Multiply(x=w842, y=2.0) -> (x*y=w821:dbl)
                              n265 = Reciprocal(x=w821) -> (1/x=w822:dbl)
                              n266 = Multiply(x=w831, y=w821) -> (x*y=w845:dbl)
                              n267 = call <vilib>:"Signal Generator by Duration.vi"("signal type"=w823, "duration"=w821, "# of samples"=w845, "frequency"=w822, "amplitude"=w837, "dc offset"=w836, "phase in"=270.0) -> ("signal"=w826:dbl[], "error"=w824:i32)  [unwired: 5 in, 2 out]
                            }
                            frame #2 {
                              # "Square Wave"
                              n268 = Select(t=-1, s=w859, f=w858) -> (s? t:f=w851:u32)
                              n269 = Reciprocal(x=w847) -> (1/x=w846:dbl)
                              n270 = Reciprocal(x=w856) -> (1/x=w850:dbl)
                              n271 = Multiply(x=w856, y=w846) -> (x*y=w861:dbl)
                              n272 = call <vilib>:"Signal Generator by Duration.vi"("signal type"=w857, "duration"=w846, "# of samples"=w861, "frequency"=w847, "amplitude"=w855, "dc offset"=w854, "phase in"=w853, "square wave duty cycle (%)"=w848) -> ("signal"=w852:dbl[], "error"=w849:i32)  [unwired: 4 in, 2 out]
                            }
                            frame #3 {
                              # "Ramp"
                              n273 = Subtract(x=w871, y=w870) -> (x-y=w874:dbl)
                              n274 = Divide(x=w874, y=w872) -> (x/y=w873:dbl)
                              n275 = Absolute Value(x=w873) -> (abs(x)=w862:dbl)
                              n276 = Reciprocal(x=w863) -> (1/x=w864:dbl)
                              n277 = Reciprocal(x=w862) -> (1/x=w865:dbl)
                              n278 = Multiply(x=w863, y=w862) -> (x*y=w876:dbl)
                              n279 = call <vilib>:"Signal Generator by Duration.vi"("signal type"=w866, "duration"=w862, "# of samples"=w876, "frequency"=w865, "amplitude"=w874, "dc offset"=w870, "phase in"=0.0) -> ("signal"=w868:dbl[], "error"=w867:i32)  [unwired: 5 in, 2 out]
                            }
                            frame #4 {
                              # "Single Point"
                              n280 = Reciprocal(x=w882) -> (1/x=w879:dbl)
                              n281 = Initialize Array(w877, 1 ("dimension size")) -> (w880:dbl[])
                            }
                            frame #5 {
                              w886 = T10 2 items=["both", "start of string", "end of string"] ("location (both)")
                              (unwired) TRUE ("convert eol (F)")
                              # "From File"
                              n282 = local read "Filename"() -> (w904:path)
                              n283 = Select(t=-1, s=w894, f=w893) -> (s? t:f=w890:u32)
                              n284 = call <vilib>:"Open_Create_Replace File.vi"("function (open:0)"=T6."open (read only)", "file path"=w904) -> ("error out"=w901:errorcluster, "file size (bytes)"=w902:i32, "new file path"=w903:path, "refnum"=w905:refnum<file>)  [unwired: 6 in]
                              n285 = local write "Filename"(w903) -> ()
                              n286 = Reciprocal(x=w892) -> (1/x=w891:dbl)
                              n287 = Read from Text File(file (use dialog)=w905, count=w902, error in=w901) -> (refnum out=w895:refnum<file>, text=w885:string, error out=w896:errorcluster)  [unwired: 1 in, 1 out]
                              n288 = local write "From File Refnum"(w895) -> ()
                              n289 = Close File(refnum=w895, error in=w896) -> ()  [unwired: 2 out]
                              n290 = call <vilib>:"Trim Whitespace.vi"("string"=w885, "location (both)"=w886) -> ("trimmed string"=w884:string)
                              n291 = local write "File Data"(w884) -> ()
                              n292 = Spreadsheet String To Array(delimiter (Tab)="\n", format string="%f", spreadsheet string=w884, array type (2D Dbl)=dbl[] [] ("initialized array")) -> (array=w889:dbl[])
                            }
                            frame #6 {
                              n293 = Reciprocal(x=w913) -> (1/x=w912:dbl)
                              n294 = Select(t=-1, s=w908, f=w907) -> (s? t:f=w906:u32)
                            }
                          }
                          n295 = call <vilib>:"Error Cluster From Error Code.vi"("error in (no error)"=w770, "error code (0)"=w791) -> ("error out"=w772:errorcluster)  [unwired: 7 in]
                          n296 = property on="Vs. T" class="WaveformChart (strict)"("X Scale.Offset and Multiplier:Multiplier"=w764, "X Scale.Range:Minimum"=0.0, "X Scale.Range:Maximum"=10.0 ("y")) -> ()  [unwired: 2 in, 2 out]
                          n297 = local read "Log Data To File"() -> (w793:bool)
                          n298 = local read "Log File Refnum"() -> (w794:refnum<file>)
                          n299 = local read "CtrlMode"() -> (w767:u32)
                          n300 = local read "GAMRYCOMLib.IGamrySignal"() -> (w786:refnum<k7>)
                          n301 = local read "CtrlMode"() -> (w773:u32)
                          n302 = local read "Pstat"() -> (w774:refnum<k7>)
                          n303 = local read "Signal"() -> (w766:refnum<k7>)
                          n304 = case shown="True" w793 {
                            tunnel: w794 -> [_ w805]
                            tunnel: [w798 w802] -> w771
                            tunnel: w762 -> [_ w801]
                            tunnel: w772 -> [w798 w800]
                            tunnel: w767 -> [_ w799]
                            frame #0 {
                            }
                            frame #1 {
                              n305 = call "Write File Header.vi"("Curve Name"="VFPCURVE", "App Name"="VFP600", "error in"=w800, "Hz"=w801, "Control Mode"=w799, "File Refnum In"=w805) -> ("error out"=w802:errorcluster)  [unwired: 2 in, 1 out]
                            }
                          }
                          n306 = call "SigArrayInit.vi"("Signal Array"=w785, "Pstat"=w774, "Signal In"=w766, "CtrlMode"=w773, "Cycles"=w795, "Sample Rate"=w764, "error in (no error)"=w771) -> ("Pstat Out"=w789:refnum<k7>, "Signal Out"=w769:refnum<k7>, "error out"=w790:errorcluster)  [unwired: 6 in]
                          n307 = Variant To Data(error in=w790, Variant=w769, type=w786) -> (error out=w788:errorcluster, data=w787:refnum<k7>)
                          n308 = invoke class="IGamryPstat" method="SetSignal"(reference=w789, error in=w788, "Signal"=w787) -> (reference out=w761:refnum<k7>, error out=w760:errorcluster)  [unwired: 1 in, 2 out]
                          n309 = invoke class="IGamryPstat" method="InitSignal"(reference=w761, error in=w760) -> (error out=w759:errorcluster)  [unwired: 1 in, 2 out]
                          n310 = case shown="No Error" w759 {
                            tunnel: [DataAcqStates."Data Acq Setup" ("Data Acq States") DataAcqStates."STOP" ("Data Acq States")] -> w768
                            frame #0 {
                            }
                            frame #1 {
                            }
                          }
                        }
                      }
                    }
                    frame #3 {
                      n311 = case shown="No Error" w917 {
                        selector: w917 -> [w928 w930]
                        tunnel: [w928 w930] -> w918
                        frame #0 {
                          w929 = TRUE ("ForcePstatFunctionUpdate")
                          n312 = property on="ForcePstatFunctionUpdate" class="Boolean (strict)"("Value (Signaling)"=w929) -> ()  [unwired: 2 in, 2 out]
                          n313 = local write "Taking Data"(w929) -> ()
                        }
                        frame #1 {
                        }
                      }
                      n314 = local read "Auto Cell Switch"() -> (w919:bool)
                      n315 = local read "Pstat"() -> (w915:refnum<k7>)
                      n316 = case shown="True" w919 {
                        tunnel: w918 -> [w922 w927]
                        tunnel: [w922 w925] -> w914
                        tunnel: w915 -> [_ w923]
                        frame #0 {
                        }
                        frame #1 {
                          w926 = 1 items=["CellOff", "CellOn"] ("CellState")
                          n317 = local write "Cell State"(TRUE) -> ()
                          n318 = invoke class="IGamryPstat" method="SetCell"(reference=w923, error in=w927, "CellState"=w926) -> (error out=w925:errorcluster)  [unwired: 1 in, 3 out]
                        }
                      }
                      n319 = case shown="No Error" w914 {
                        tunnel: [DataAcqStates."Acquire Data" ("Data Acq States") DataAcqStates."STOP" ("Data Acq States")] -> w916
                        frame #0 {
                        }
                        frame #1 {
                        }
                      }
                    }
                    frame #4 {
                      # "Tell the Dtaq to Run"
                      n320 = local read "Dtaq"() -> (w934:refnum<k7>)
                      n321 = invoke class="IGamryDtaqIv" method="Run"(reference=w934, error in=w933, "AutoRun"=TRUE) -> (error out=w936:errorcluster)  [unwired: 1 in, 3 out]
                      n322 = while {
                        tunnel: [w958] -> w931
                        tunnel: w936 -> [w961]
                        stop <- w963 stop-if-true
                        # "Overload"
                        # "If we fail here, it is likely due to a device being turned off,\nas any \"Dtaq not initialized\" errors would crop up in earlier states,\nso we'll give a more helpful error."
                        # "Im"
                        # "Vf"
                        # "Take the actual data"
                        # "Poll 2x as often as axq frequency, or X ms, whichever is larger."
                        n323 = local read "Acq. Frequency"() -> (w977:dbl)
                        n324 = local read "Dtaq"() -> (w982:refnum<k7>)
                        n325 = invoke class="IGamryDtaqIv" method="Cook"(reference=w982, error in=w961, "NumPoints"=1024) -> (error out=w959:errorcluster, "Data"=w980:variant)  [unwired: 2 in, 3 out]
                        n326 = local read "Im History"() -> (w953:sgl[])
                        n327 = local read "Vf History"() -> (w956:sgl[])
                        n328 = Reciprocal(x=w977) -> (1/x=w976:dbl)
                        n329 = Multiply(x=w976, y=1000.0) -> (x*y=w974:dbl)
                        n330 = Divide(x=w974, y=2.0) -> (x/y=w972:dbl)
                        n331 = Array Size(array=w953) -> (size(s)=w949:i32)
                        n332 = Array Size(array=w956) -> (size(s)=w967:i32)
                        n333 = Subtract(x=w949, y=16384) -> (x-y=w951:i32)
                        n334 = Max & Min(x=w972, y=60.0) -> (max(x,y)=w970:dbl)  [unwired: 1 out]
                        n335 = Subtract(x=w967, y=16384) -> (x-y=w965:i32)
                        n336 = Array Subset(array=w953, index=w951) -> (w952:sgl[])  [unwired: 1 in]
                        n337 = Array Subset(array=w956, index=w965) -> (w962:sgl[])  [unwired: 1 in]
                        n338 = Variant To Data(error in=w959, Variant=w980, type=sgl[][] []) -> (error out=w939:errorcluster, data=w941:sgl[][])
                        n339 = Wait (ms)(milliseconds to wait=w970) -> ()  [unwired: 1 out]
                        n340 = Index Array(array=w941, index (row)=1) -> (element=w955:sgl[])  [unwired: 1 in]
                        n341 = Index Array(array=w941, index (row)=3) -> (element=w948:sgl[])  [unwired: 1 in]
                        n342 = Index Array(array=w941, index (row)=5) -> (element=w940:sgl[])  [unwired: 1 in]
                        n343 = Build Array(w955, w948) -> (w954:sgl[][])
                        n344 = Build Array (concatenate)(w952, w948) -> (w946:sgl[])
                        n345 = Build Array (concatenate)(w962, w955) -> (w947:sgl[])
                        n346 = local write "Vs. T"(w954) -> ()
                        n347 = local write "Im History"(w946) -> ()
                        n348 = local read "XY Graph Flipped?"() -> (w944:bool)
                        n349 = local write "Vf History"(w947) -> ()
                        n350 = for {
                          tunnel: w940 -> [w998] mode=indexing
                          w986 = cluster{u32, u32}[] [{7536640, 7536640}, {16744448, 16744448}]
                          w987 = cluster{u32, u32}[] [{7536640, 7536640}, {16711680, 16711680}]
                          n351 = call "VFPOverloads.vi"("Overload IN"=w998) -> ("Overloads"=w992:T11)  [unwired: 9 in, 1 out]
                          n352 = Unbundle By Name(w992) -> ("CA Overload"=w996:bool)
                          n353 = Unbundle By Name(w992) -> ("I Overload"=w988:bool, "I ADC Railed"=w991:bool)
                          n354 = Unbundle By Name(w992) -> ("V Overload"=w994:bool, "V ADC Railed"=w993:bool)
                          n355 = Or(x=w988, y=w991) -> (x .or. y?=w990:bool)
                          n356 = Or(x=w994, y=w993) -> (x .or. y?=w995:bool)
                          n357 = local write "Control Amp Overload"(w996) -> ()
                          n358 = Select(t=w987, s=w994, f=w986) -> (s? t:f=w997:cluster{u32, u32}[])
                          n359 = Select(t=w987, s=w988, f=w986) -> (s? t:f=w989:cluster{u32, u32}[])
                          n360 = property on="Voltage Overload" class="Boolean (strict)"("Value"=w995, "Colors [4]"=w997) -> ()  [unwired: 2 in, 2 out]
                          n361 = property on="Current Overload" class="Boolean (strict)"("Value"=w990, "Colors [4]"=w989) -> ()  [unwired: 2 in, 2 out]
                        }
                        n362 = case shown="False" w944 {
                          tunnel: w947 -> [w1001 w1004]
                          tunnel: w946 -> [w1000 w1003]
                          tunnel: [w999 w1002] -> w945
                          frame #0 {
                            n363 = Build Cluster Array(w1000, w1001) -> (w999:cluster{sgl, sgl}[])
                          }
                          frame #1 {
                            n364 = Build Cluster Array(w1004, w1003) -> (w1002:cluster{sgl, sgl}[])
                          }
                        }
                        n365 = local read "DataDone?"() -> (w983:bool)
                        n366 = local read "Start/Stop"() -> (w985:bool)
                        n367 = local write "I vs. V"(w945) -> ()
                        n368 = Not(x=w985) -> (.not. x?=w984:bool)
                        n369 = call <vilib>:"Find First Error.vi"("error in (no error)"=w939) -> ("error out"=w957:errorcluster, "error?"=w960:bool)  [unwired: 3 in]
                        n370 = Or(x=w983, y=w984) -> (x .or. y?=w964:bool)
                        n371 = Or(x=w960, y=w964) -> (x .or. y?=w963:bool)
                        n372 = local read "Log Data To File"() -> (w969:bool)
                        n373 = local read "Log File Refnum"() -> (w968:refnum<file>)
                        n374 = case shown="No Error" w957 {
                          selector: w957 -> [w1005 w1007]
                          tunnel: [w1005 w1006] -> w958
                          frame #0 {
                          }
                          frame #1 {
                            n375 = Bundle By Name(cluster=w1007, "source"="Data Acq\n\nPlease confirm that your device has \nnot been disabled or disconnected.") -> (w1006:errorcluster)
                          }
                        }
                        n376 = case shown="True" w969 {
                          tunnel: w968 -> [_ w1014]
                          tunnel: w954 -> [_ w1010]
                          frame #0 {
                          }
                          frame #1 {
                            n377 = Transpose 2D Array(2D array=w1010) -> (transposed array=w1011:sgl[][])
                            n378 = Array To Spreadsheet String(array=w1011, 3:"%5g" ("format string")) -> (spreadsheet string=w1013:string)  [unwired: 1 in]
                            n379 = Write to Binary File(file (use dialog)=w1014, data=w1013, 5:FALSE ("prepend array or string size? (T)")) -> ()  [unwired: 3 in, 3 out]
                          }
                        }
                      }
                      n380 = case shown="No Error" w931 {
                        tunnel: [DataAcqStates."Cleanup" ("Data Acq States") DataAcqStates."STOP" ("Data Acq States")] -> w932
                        frame #0 {
                        }
                        frame #1 {
                        }
                      }
                    }
                    frame #5 {
                      n381 = local read "Auto Cell Switch"() -> (w1024:bool)
                      n382 = local read "Device Gone"() -> (w1022:bool)
                      n383 = Not(x=w1022) -> (.not. x?=w1025:bool)
                      n384 = local read "Pstat"() -> (w1020:refnum<k7>)
                      n385 = And(x=w1024, y=w1025) -> (x .and. y?=w1026:bool)
                      n386 = case shown="True" w1026 {
                        tunnel: [w1040 w1045] -> w1027
                        tunnel: w1021 -> [w1040 w1043]
                        tunnel: w1020 -> [_ w1042]
                        frame #0 {
                        }
                        frame #1 {
                          w1041 = 0 items=["CellOff", "CellOn"] ("CellState")
                          n387 = invoke class="IGamryPstat" method="SetCell"(reference=w1042, error in=w1043, "CellState"=w1041) -> (error out=w1045:errorcluster)  [unwired: 1 in, 3 out]
                          n388 = local write "Cell State"(FALSE) -> ()
                        }
                      }
                      n389 = local read "Dtaq"() -> (w1023:refnum<k7>)
                      n390 = invoke class="IGamryDtaqIv" method="Stop"(reference=w1023, error in=w1027) -> (reference out=w1017:refnum<k7>, error out=w1016:errorcluster)  [unwired: 1 in, 1 out]
                      n391 = while {
                        shift-right: [w1029] -> _
                        shift-left: w1017 -> [w1034]
                        shift-right: [w1030] -> w1015
                        shift-left: w1016 -> [w1033]
                        stop <- w1031 stop-if-true
                        n392 = invoke class="IGamryDtaqIv" method="Cook"(reference=w1034, error in=w1033, "NumPoints"=1024) -> (reference out=w1029:refnum<k7>, error out=w1030:errorcluster, "NumPoints"=w1032:i32)  [unwired: 2 in, 2 out]
                        n393 = Equal To 0?(x=w1032) -> (x = 0?=w1031:bool)
                      }
                      n394 = case shown="No Error" w1015 {
                        selector: w1015 -> [w1036 w1037]
                        tunnel: [w1036 w1037] -> w1018
                        frame #0 {
                          n395 = local write "Taking Data"(FALSE) -> ()
                        }
                        frame #1 {
                        }
                      }
                      n396 = case shown="No Error" w1018 {
                        tunnel: [DataAcqStates."STOP" ("Data Acq States") DataAcqStates."STOP" ("Data Acq States")] -> w1019
                        frame #0 {
                        }
                        frame #1 {
                        }
                      }
                    }
                    frame #6 {
                      w1051 = u8 0 ("Disabled")
                      w1046 = FALSE
                      w1054 = FALSE ("Begin")
                      # "Enable menu items"
                      # "Reset Buttons"
                      n397 = property class="App"() -> ("Application:Kind"=w1052:T12)  [unwired: 2 in, 2 out]
                      n398 = local read "Log Data To File"() -> (w1061:bool)
                      n399 = case shown="\"Run Time System\", Default" w1052 {
                        tunnel: [w1064 w1065] -> w1053
                        frame #0 {
                          w1064 = T13 1 items=["no dialog", "OK message", "continue or stop message", "OK message + warnings", "continue/stop + warnings"] ("type of dialog (OK msg:1)")
                        }
                        frame #1 {
                          w1065 = T13 1 items=["no dialog", "OK message", "continue or stop message", "OK message + warnings", "continue/stop + warnings"] ("type of dialog (OK msg:1)")
                        }
                      }
                      n400 = local read "[user-defined descriptions]"() -> (w1055:string[])
                      n401 = local write "Start/Stop"(w1054) -> ()
                      n402 = local write "DataDone?"(w1054) -> ()
                      n403 = local write "Device Gone"(w1054) -> ()
                      n404 = local read "[user-defined codes]"() -> (w1047:u32[])
                      n405 = case shown="True" w1061 {
                        tunnel: [w1070 w1072] -> w1058
                        tunnel: w1057 -> [w1070 w1071]
                        frame #0 {
                        }
                        frame #1 {
                          n406 = local read "Log File Refnum"() -> (w1073:refnum<file>)
                          n407 = Close File(refnum=w1073, error in=w1071) -> (error out=w1072:errorcluster)  [unwired: 1 out]
                        }
                      }
                      n408 = local read "DataDone Callback"() -> (w1059:refnum<k27>)
                      n409 = local write "Control Amp Overload"(w1046) -> ()
                      n410 = local write "Voltage Overload"(w1046) -> ()
                      n411 = local write "Current Overload"(w1046) -> ()
                      n412 = Not A Number/Path/Refnum?(number/path/refnum=w1059) -> (NaN/Path/Refnum?=w1060:bool)
                      n413 = case shown="False" w1060 {
                        tunnel: w1059 -> [w1068 _]
                        tunnel: w1058 -> [w1067 w1069]
                        tunnel: [w1066 w1069] -> w1049
                        frame #0 {
                          n414 = Unregister For Events(event registration refnum=w1068, error in=w1067) -> (error out=w1066:errorcluster)
                        }
                        frame #1 {
                        }
                      }
                      n415 = property on="Device" class="Ring (strict)"("Disabled"=w1051) -> ()  [unwired: 2 in, 2 out]
                      n416 = property on="CtrlMode" class="Ring (strict)"("Disabled"=w1051) -> ()  [unwired: 2 in, 2 out]
                      n417 = property on="Acq. Frequency" class="DigNum (strict)"("Disabled"=w1051) -> ()  [unwired: 2 in, 2 out]
                      n418 = call <vilib>:"General Error Handler.vi"("[user-defined codes]"=w1047, "[user-defined descriptions]"=w1055, "type of dialog (OK msg:1)"=w1053, "error in (no error)"=w1049) -> ("error out"=w1048:errorcluster)  [unwired: 7 in, 4 out]
                      n419 = property on="Vch Range" class="Ring (strict)"("Disabled"=w1051) -> ()  [unwired: 2 in, 2 out]
                      n420 = property on="Ich Range" class="Ring (strict)"("Disabled"=w1051) -> ()  [unwired: 2 in, 2 out]
                      n421 = property on="Log Data To File" class="Boolean (strict)"("Disabled"=w1051) -> ()  [unwired: 2 in, 2 out]
                      n422 = local read "CtrlMode"() -> (w1050:u32)
                      n423 = case shown="1, Default" w1050 {
                        frame #0 {
                          w1062 = u8 0 ("Disabled")
                          n424 = property on="I/E Range" class="Ring (strict)"("Disabled"=w1062) -> ()  [unwired: 2 in, 2 out]
                          n425 = property on="I/E Autorange" class="Bool (strict)"("Disabled"=w1062) -> ()  [unwired: 2 in, 2 out]
                        }
                        frame #1 {
                          w1063 = u8 2 ("Disabled")
                          n426 = property on="I/E Range" class="Ring (strict)"("Disabled"=w1063) -> ()  [unwired: 2 in, 2 out]
                          n427 = property on="I/E Autorange" class="Bool (strict)"("Disabled"=w1063) -> ()  [unwired: 2 in, 2 out]
                        }
                      }
                    }
                  }
                  n428 = Equal?(x=w665, y=DataAcqStates."STOP" ("Data Acq States")) -> (x = y?=w666:bool)
                  n429 = Wait (ms)(milliseconds to wait=u32 150) -> ()  [unwired: 1 out]
                }
              }
            }
          }
          event #1 {
            n430 = event-data() -> ()  [unwired: 1 in, 3 out]
          }
        }
        n431 = local read "Close"() -> (w656:bool)
        n432 = Not(x=w656) -> (.not. x?=w655:bool)
      }
      n433 = while {
        stop <- w164 continue-if-true
        n434 = local read "milliseconds to wait"() -> (w163:u32)
        n435 = event shown="[0] Timeout" {
          selector: _ -> [_ _ _ _ _ _ _ _]
          dyn-events: _ -> [_ _ _ _ _ _ _ _]
          timeout: w163 -> [_ _ _ _ _ _ _ _]
          event #0 {
            w167 = u32 2 items=["Galvanostat", "Potentiostat", "ZRA"] ("CtrlMode")
            n436 = event-data() -> ()  [unwired: 1 in, 2 out]
            n437 = local read "Taking Data"() -> (w176:bool)
            n438 = case shown="True" w176 {
              frame #0 {
              }
              frame #1 {
                n439 = local read "Pstat"() -> (w177:refnum<k7>)
                n440 = local read "Vch Autorange"() -> (w179:bool)
                n441 = local read "Ich Autorange"() -> (w180:bool)
                n442 = local read "I/E Autorange"() -> (w178:bool)
                n443 = case shown="False" w180 {
                  tunnel: w177 -> [_ w201]
                  frame #0 {
                    n444 = property on="Ich Range" class="Ring (strict)"("Disabled"=0) -> ()  [unwired: 2 in, 2 out]
                  }
                  frame #1 {
                    n445 = invoke class="IGamryPstat" method="IchRange"(reference=w201) -> ("IchRange"=w200:i32)  [unwired: 2 in, 2 out]
                    n446 = property on="Ich Range" class="Ring (strict)"("Value"=w200, "Disabled"=1) -> ()  [unwired: 2 in, 2 out]
                  }
                }
                n447 = case shown="False" w179 {
                  tunnel: w177 -> [_ w197]
                  frame #0 {
                    n448 = property on="Vch Range" class="Ring (strict)"("Disabled"=0) -> ()  [unwired: 2 in, 2 out]
                  }
                  frame #1 {
                    n449 = invoke class="IGamryPstat" method="VchRange"(reference=w197) -> ("VchRange"=w196:i32)  [unwired: 2 in, 2 out]
                    n450 = property on="Vch Range" class="Ring (strict)"("Value"=w196, "Disabled"=1) -> ()  [unwired: 2 in, 2 out]
                  }
                }
                n451 = case shown="False" w178 {
                  tunnel: w177 -> [_ w193]
                  frame #0 {
                    n452 = local read "CtrlMode"() -> (w181:u32)
                    n453 = case shown="1, Default" w181 {
                      frame #0 {
                        w182 = u8 0 ("Disabled")
                        n454 = property on="I/E Range" class="Ring (strict)"("Disabled"=w182) -> ()  [unwired: 2 in, 2 out]
                        n455 = property on="I/E Autorange" class="Bool (strict)"("Disabled"=w182) -> ()  [unwired: 2 in, 2 out]
                      }
                      frame #1 {
                        w183 = u8 2 ("Disabled")
                        n456 = property on="I/E Range" class="Ring (strict)"("Disabled"=w183) -> ()  [unwired: 2 in, 2 out]
                        n457 = property on="I/E Autorange" class="Bool (strict)"("Disabled"=w183) -> ()  [unwired: 2 in, 2 out]
                      }
                    }
                  }
                  frame #1 {
                    w188 = u32 0 items=["Galvanostat", "Potentiostat", "ZRA"] ("CtrlMode")
                    n458 = invoke class="IGamryPstat" method="IERange"(reference=w193) -> ("IERange"=w191:i32)  [unwired: 2 in, 2 out]
                    n459 = local read "CtrlMode"() -> (w189:u32)
                    n460 = local read "First I/E Range"() -> (w190:i32)
                    n461 = Equal?(x=w189, y=w188) -> (x = y?=w187:bool)
                    n462 = Select(t=2, s=w187, f=1) -> (s? t:f=w184:i32)
                    n463 = Subtract(x=w191, y=w190) -> (x-y=w192:i32)
                    n464 = property on="I/E Range" class="Ring (strict)"("Value"=w192, "Disabled"=w184) -> ()  [unwired: 2 in, 2 out]
                  }
                }
              }
            }
            n465 = local read "CtrlMode"() -> (w166:u32)
            n466 = local read "Family"() -> (w168:string)
            n467 = Equal?(x=w166, y=w167) -> (x = y?=w170:bool)
            n468 = Equal?(x=w168, y="PC5") -> (x = y?=w171:bool)
            n469 = And(x=w170, y=w171) -> (x .and. y?=w172:bool)
            n470 = Select(t=i32[] [0], s=w172, f=i32[] []) -> (s? t:f=w174:i32[])
            n471 = property on="CA Speed" class="Ring (strict)"("Disabled Items []"=w174) -> ()  [unwired: 2 in, 2 out]
          }
          event #1 {
            n472 = event-data() -> ("NewVal"=w202:u16)  [unwired: 1 in]
            n473 = case shown="2" w202 {
              frame #0 {
                n474 = property on="Vs. T" class="WaveformChart (strict)"("Visible"=TRUE) -> ()  [unwired: 2 in, 2 out]
                n475 = property on="I vs. V" class="XYGraph (strict)"("Visible"=FALSE) -> ()  [unwired: 2 in, 2 out]
              }
              frame #1 {
                n476 = property on="Vs. T" class="WaveformChart (strict)"("Visible"=FALSE) -> ()  [unwired: 2 in, 2 out]
                n477 = local write "XY Graph Flipped?"(FALSE ("XY Graph Flipped?")) -> ()
                n478 = local read "Taking Data"() -> (w205:bool)
                n479 = case shown="False" w205 {
                  frame #0 {
                    n480 = local read "Im History"() -> (w214:sgl[])
                    n481 = local read "Vf History"() -> (w215:sgl[])
                    n482 = Build Cluster Array(w215, w214) -> (w213:cluster{sgl, sgl}[])
                    n483 = local write "I vs. V"(w213) -> ()
                  }
                  frame #1 {
                  }
                }
                n484 = property on="I vs. V" class="XYGraph (strict)"("Visible"=TRUE, "X Scale.Name Label.Text"="Voltage (V)", "Y Scale.Name Label.Text"="Current (A)", "Transpose Array"=FALSE, "Plot.Plot Name"="I vs. V") -> ()  [unwired: 2 in, 2 out]
              }
              frame #2 {
                n485 = property on="Vs. T" class="WaveformChart (strict)"("Visible"=FALSE) -> ()  [unwired: 2 in, 2 out]
                n486 = local write "XY Graph Flipped?"(TRUE ("XY Graph Flipped?")) -> ()
                n487 = local read "Taking Data"() -> (w216:bool)
                n488 = case shown="False" w216 {
                  frame #0 {
                    n489 = local read "Im History"() -> (w225:sgl[])
                    n490 = local read "Vf History"() -> (w226:sgl[])
                    n491 = Build Cluster Array(w225, w226) -> (w224:cluster{sgl, sgl}[])
                    n492 = local write "I vs. V"(w224) -> ()
                  }
                  frame #1 {
                  }
                }
                n493 = property on="I vs. V" class="XYGraph (strict)"("Visible"=TRUE, "X Scale.Name Label.Text"="Current (A)", "Y Scale.Name Label.Text"="Voltage (V)", "Transpose Array"=FALSE, "Plot.Plot Name"="V vs. I") -> ()  [unwired: 2 in, 2 out]
              }
            }
          }
          event #2 {
            n494 = event-data() -> ("NewVal"=w228:bool)  [unwired: 1 in, 5 out]
            n495 = local read "Device Open"() -> (w227:bool)
            n496 = case shown="True" w227 {
              tunnel: w228 -> [_ w231]
              frame #0 {
              }
              frame #1 {
                # "Monitor Cell Switch"
                n497 = local read "Pstat"() -> (w233:refnum<k7>)
                n498 = Boolean To (0,1)(Boolean=w231) -> (0, 1=w232:i16)
                n499 = invoke class="IGamryPstat" method="SetCell"(reference=w233, "CellState"=w232) -> ("SetCell"=w229:i32)  [unwired: 2 in, 3 out]
                n500 = Not Equal To 0?(x=w229) -> (x != 0?=→"SetCell":bool)
                "Cell Val Change NewVal" <- w231
              }
            }
          }
          event #3 {
            # "Adjust unit labels\naccording to\nControl Mode"
            n501 = event-data() -> ("CtlRef"=w235:refnum<vi>)  [unwired: 1 in]
            n502 = local read "CtrlMode"() -> (w238:u32)
            n503 = control-ref of="CtrlMode"() -> (w237:refnum<vi>)
            n504 = local read "Device Open"() -> (w243:bool)
            n505 = local read "Pstat"() -> (w242:refnum<k7>)
            n506 = To More Generic Class(target class=w235, reference=w237) -> (generic class reference=w236:refnum<vi>)
            n507 = Equal?(x=w235, y=w236) -> (x = y?=w239:bool)
            n508 = case shown="True" w239 {
              tunnel: w238 -> [_ w247]
              tunnel: [errorcluster {"status"=FALSE, "code"=0, "source"=""} ("error out") w246] -> w234
              frame #0 {
              }
              frame #1 {
                n509 = case shown="1, Default" w247 {
                  selector: w247 -> [_ w262]
                  tunnel: [w248 w267] -> w246
                  frame #0 {
                    w249 = u8 2 ("Disabled")
                    w251 = u16 0 items=["Fast", "Medium Fast", "Normal", "Slow"] ("I/E Stability")
                    w253 = "A" ("Caption.Text")
                    n510 = property on="Amplitude" class="Digital (strict)"("Caption.Text"=w253) -> ()  [unwired: 2 in, 2 out]
                    n511 = property on="Scan Rate" class="Digital (strict)"("Caption.Text"="A/s") -> ()  [unwired: 2 in, 2 out]
                    n512 = property on="DC Offset" class="Digital (strict)"("Caption.Text"=w253) -> ()  [unwired: 2 in, 2 out]
                    n513 = property on="Final" class="Digital (strict)"("Caption.Text"=w253) -> ()  [unwired: 2 in, 2 out]
                    n514 = property on="Initial" class="DigNum (strict)"("Caption.Text"=w253) -> ()  [unwired: 2 in, 2 out]
                    n515 = property on="I/E Stability" class="Ring (strict)"("Disabled"=u8 2, "Value"=w251) -> ()  [unwired: 2 in, 2 out]
                    n516 = property on="I/E Range" class="Ring (strict)"("Disabled"=w249) -> ()  [unwired: 2 in, 2 out]
                    n517 = property on="I/E Autorange" class="Bool (strict)"("Disabled"=w249, "Value"=TRUE) -> (error out=w248:errorcluster)  [unwired: 2 in, 1 out]
                  }
                  frame #1 {
                    w264 = u32 2 items=["Galvanostat", "Potentiostat", "ZRA"] ("CtrlMode")
                    w268 = u8 0 ("Disabled")
                    w270 = "V" ("Caption.Text")
                    n518 = local read "CA Speed"() -> (w256:u16)
                    n519 = local read "Family"() -> (w265:string)
                    n520 = Equal?(x=w262, y=w264) -> (x = y?=w263:bool)
                    n521 = Equal?(x=w265, y="PC5") -> (x = y?=w261:bool)
                    n522 = Equal?(x=w256, y=u16 0) -> (x = y?=w259:bool)
                    n523 = Compound Arithmetic op=AND(w263, w261, w259) -> (w258:bool)
                    n524 = Select(t=u16 1, s=w258, f=w256) -> (s? t:f=w257:u16)
                    n525 = local write "CA Speed"(w257) -> ()
                    n526 = property on="Amplitude" class="Digital (strict)"("Caption.Text"=w270) -> ()  [unwired: 2 in, 2 out]
                    n527 = property on="Scan Rate" class="Digital (strict)"("Caption.Text"="V/s") -> ()  [unwired: 2 in, 2 out]
                    n528 = property on="DC Offset" class="Digital (strict)"("Caption.Text"=w270) -> ()  [unwired: 2 in, 2 out]
                    n529 = property on="Final" class="Digital (strict)"("Caption.Text"=w270) -> ()  [unwired: 2 in, 2 out]
                    n530 = property on="Initial" class="DigNum (strict)"("Caption.Text"=w270) -> ()  [unwired: 2 in, 2 out]
                    n531 = property on="I/E Stability" class="Ring (strict)"("Disabled"=u8 0) -> ()  [unwired: 2 in, 2 out]
                    n532 = property on="I/E Range" class="Ring (strict)"("Disabled"=w268) -> ()  [unwired: 2 in, 2 out]
                    n533 = property on="I/E Autorange" class="Bool (strict)"("Disabled"=w268) -> (error out=w267:errorcluster)  [unwired: 2 in, 1 out]
                  }
                }
              }
            }
            n534 = case shown="True" w243 {
              tunnel: w242 -> [_ w278]
              tunnel: [errorcluster {"status"=FALSE, "code"=0, "source"=""} ("error out") w285] -> w240
              tunnel: w234 -> [_ w274]
              frame #0 {
              }
              frame #1 {
                w317 = 0 items=["StabilityFast", "StabilityMedFast", "StabilityNorm", "StabilitySlow"] ("Stability")
                w320 = 0 items=["GstatMode", "PstatMode", "ZRAMode", "FRAMode"] ("SetCtrlMode")
                n535 = local read "CtrlMode"() -> (w338:u32)
                n536 = local read "Ich Autorange"() -> (w327:bool)
                n537 = local read "IchOffsetEnable"() -> (w309:bool)
                n538 = local read "Ich Filter"() -> (w305:u16)
                n539 = local read "Ich Range"() -> (w336:u16)
                n540 = invoke class="IGamryPstat" method="SetCtrlMode"(reference=w278, error in=w274, "CtrlMode"=w338) -> (reference out=w314:refnum<k7>, error out=w315:errorcluster, "SetCtrlMode"=w319:i32)  [unwired: 1 in, 1 out]
                n541 = invoke class="IGamryPstat" method="SetIchFilter"(reference=w278, "Filter"=w305) -> (reference out=w302:refnum<k7>, error out=w301:errorcluster, "SetIchFilter"=w306:i32)  [unwired: 2 in, 1 out]
                n542 = invoke class="IGamryPstat" method="SetIchRange"(reference=w278, "Range"=w336) -> (reference out=w297:refnum<k7>, error out=w298:errorcluster, "SetIchRange"=w337:i32)  [unwired: 2 in, 1 out]
                n543 = invoke class="IGamryPstat" method="SetIchRangeMode"(reference=w278, "RangeMode"=w327) -> (reference out=w293:refnum<k7>, error out=w294:errorcluster, "SetIchRangeMode"=w328:bool)  [unwired: 2 in, 1 out]
                n544 = invoke class="IGamryPstat" method="SetIchOffsetEnable"(reference=w278, "OffsetEnable"=w309) -> (reference out=w299:refnum<k7>, error out=w300:errorcluster, "SetIchOffsetEnable"=w310:bool)  [unwired: 2 in, 1 out]
                n545 = local write "CtrlMode"(w319) -> ()
                n546 = local write "Ich Autorange"(w328) -> ()
                n547 = local write "IchOffsetEnable"(w310) -> ()
                n548 = local write "Ich Range"(w337) -> ()
                n549 = local write "Ich Filter"(w306) -> ()
                n550 = local read "I/E Stability"() -> (w318:u16)
                n551 = local read "Vch Range"() -> (w334:u16)
                n552 = local read "Vch Autorange"() -> (w325:bool)
                n553 = local read "Vch Filter"() -> (w304:u16)
                n554 = local read "VchOffsetEnable"() -> (w307:bool)
                n555 = Equal?(x=w319, y=w320) -> (x = y?=w321:bool)
                n556 = invoke class="IGamryPstat" method="SetVchFilter"(reference=w302, error in=w301, "Filter"=w304) -> (error out=w288:errorcluster, "SetVchFilter"=w303:i32)  [unwired: 1 in, 2 out]
                n557 = invoke class="IGamryPstat" method="SetVchRange"(reference=w297, error in=w298, "Range"=w334) -> (reference out=w295:refnum<k7>, error out=w296:errorcluster, "SetVchRange"=w335:i32)  [unwired: 1 in, 1 out]
                n558 = invoke class="IGamryPstat" method="SetVchRangeMode"(reference=w293, error in=w294, "RangeMode"=w325) -> (reference out=w291:refnum<k7>, error out=w292:errorcluster, "SetVchRangeMode"=w326:bool)  [unwired: 1 in, 1 out]
                n559 = Select(t=w317, s=w321, f=w318) -> (s? t:f=w316:i32)
                n560 = local write "Vch Range"(w335) -> ()
                n561 = local write "Vch Autorange"(w326) -> ()
                n562 = local write "Vch Filter"(w303) -> ()
                n563 = invoke class="IGamryPstat" method="SetVchOffsetEnable"(reference=w299, error in=w300, "OffsetEnable"=w307) -> (reference out=w277:refnum<k7>, error out=w276:errorcluster, "SetVchOffsetEnable"=w308:bool)  [unwired: 1 in, 1 out]
                n564 = invoke class="IGamryPstat" method="SetIEStability"(reference=w314, error in=w315, "Stability"=w316) -> (reference out=w311:refnum<k7>, error out=w312:errorcluster, "SetIEStability"=w322:i32)  [unwired: 1 in, 1 out]
                n565 = local write "VchOffsetEnable"(w308) -> ()
                n566 = local write "I/E Stability"(w322) -> ()
                n567 = local read "I/E Range"() -> (w329:u16)
                n568 = local read "First I/E Range"() -> (w330:i32)
                n569 = local read "I/E Autorange"() -> (w323:bool)
                n570 = local read "Ich Offset"() -> (w283:sgl)
                n571 = local read "CA Speed"() -> (w273:u16)
                n572 = Add(x=w329, y=w330) -> (x+y=w332:i32)
                n573 = invoke class="IGamryPstat" method="SetIERangeMode"(reference=w291, error in=w292, "RangeMode"=w323) -> (error out=w286:errorcluster, "SetIERangeMode"=w324:bool)  [unwired: 1 in, 2 out]
                n574 = local write "I/E Autorange"(w324) -> ()
                n575 = invoke class="IGamryPstat" method="SetIERange"(reference=w295, error in=w296, "Range"=w332) -> (error out=w287:errorcluster, "SetIERange"=w333:i32)  [unwired: 1 in, 2 out]
                n576 = invoke class="IGamryPstat" method="SetIchOffset"(reference=w277, error in=w276, "Offset"=w283) -> (reference out=w280:refnum<k7>, error out=w279:errorcluster, "SetIchOffset"=w284:sgl)  [unwired: 1 in, 1 out]
                n577 = invoke class="IGamryPstat" method="SetCASpeed"(reference=w311, error in=w312, "CASpeed"=w273) -> (error out=w289:errorcluster, "SetCASpeed"=w313:i32)  [unwired: 1 in, 2 out]
                n578 = local write "Ich Offset"(w284) -> ()
                n579 = local write "CA Speed"(w313) -> ()
                n580 = Subtract(x=w333, y=w330) -> (x-y=w331:i32)
                n581 = local read "Vch Offset"() -> (w282:sgl)
                n582 = local write "I/E Range"(w331) -> ()
                n583 = invoke class="IGamryPstat" method="SetVchOffset"(reference=w280, error in=w279, "Offset"=w282) -> (error out=w275:errorcluster, "SetVchOffset"=w281:sgl)  [unwired: 1 in, 2 out]
                n584 = local write "Vch Offset"(w281) -> ()
                n585 = Build Array(w289, w288, w275, w287, w286) -> (w290:errorcluster[])
                n586 = call <vilib>:"Merge Errors.vi"("error array in"=w290) -> ("error out"=w285:errorcluster)  [unwired: 6 in]
              }
            }
            n587 = Unbundle By Name(w240) -> ("status"=w241:bool)
            n588 = local write "ForcePstatFunctionUpdate"(FALSE ("ForcePstatFunctionUpdate")) -> ()
            n589 = call "Pstat Settings Error"("Enable"=w241) -> ()  [unwired: 9 in, 2 out]
          }
          event #4 {
            # "Signal Tweak Loop"
            n590 = event-data() -> ("OldVal"=w341:variant, "NewVal"=w340:variant, "CtlRef"=w339:refnum<vi>)  [unwired: 1 in]
            n591 = local read "Continuous"() -> (w342:bool)
            n592 = local read "Signal Type"() -> (w347:u16)
            n593 = local read "Taking Data"() -> (w346:bool)
            n594 = Select(t=2, s=w342, f=0) -> (s? t:f=w343:i32)
            n595 = property on="Cycles" class="DigNum (strict)"("Disabled"=w343) -> ()  [unwired: 2 in, 2 out]
            n596 = stacked-sequence {
              tunnel: w347 -> [w348 w379]
              tunnel: w346 -> [_ w378]
              tunnel: w341 -> [_ w377]
              tunnel: w340 -> [_ w376]
              tunnel: w339 -> [_ w375]
              frame #0 {
                # "Adjust front panel according to signal type"
                n597 = case shown="3" w348 {
                  frame #0 {
                    w350 = FALSE ("Visible")
                    (unwired) FALSE ("Visible")
                    w352 = TRUE ("Visible")
                    n598 = property on="Signal Frequency" class="Digital (strict)"("Visible"=w352) -> ()  [unwired: 2 in, 2 out]
                    n599 = property on="Amplitude" class="Digital (strict)"("Visible"=w352) -> ()  [unwired: 2 in, 2 out]
                    n600 = property on="DC Offset" class="Digital (strict)"("Visible"=w352) -> ()  [unwired: 2 in, 2 out]
                    n601 = property on="Phase Offset" class="Digital (strict)"("Visible"=w352) -> ()  [unwired: 2 in, 2 out]
                    n602 = property on="Acq. Frequency" class="Digital (strict)"("Visible"=w352) -> ()  [unwired: 2 in, 2 out]
                    n603 = property on="Cycles" class="DigNum (strict)"("Visible"=w352) -> ()  [unwired: 2 in, 2 out]
                    n604 = property on="Continuous" class="Boolean (strict)"("Visible"=w352) -> ()  [unwired: 2 in, 2 out]
                    n605 = property on="Duty Cycle" class="DigNum (strict)"("Visible"=FALSE) -> ()  [unwired: 2 in, 2 out]
                    n606 = property on="Filename" class="Path"("Visible"=FALSE) -> ()  [unwired: 2 in, 2 out]
                    n607 = property on="Final" class="Digital (strict)"("Visible"=w350) -> ()  [unwired: 2 in, 2 out]
                    n608 = property on="Initial" class="Digital (strict)"("Visible"=w350) -> ()  [unwired: 2 in, 2 out]
                    n609 = property on="Scan Rate" class="Digital (strict)"("Visible"=w350) -> ()  [unwired: 2 in, 2 out]
                  }
                  frame #1 {
                    w354 = TRUE ("Visible")
                    (unwired) FALSE ("Visible")
                    w355 = FALSE ("Visible")
                    # "Triangle"
                    n610 = property on="Signal Frequency" class="Digital (strict)"("Visible"=w355) -> ()  [unwired: 2 in, 2 out]
                    n611 = property on="Amplitude" class="Digital (strict)"("Visible"=w355) -> ()  [unwired: 2 in, 2 out]
                    n612 = property on="DC Offset" class="Digital (strict)"("Visible"=w355) -> ()  [unwired: 2 in, 2 out]
                    n613 = property on="Phase Offset" class="Digital (strict)"("Visible"=w355) -> ()  [unwired: 2 in, 2 out]
                    n614 = property on="Duty Cycle" class="DigNum (strict)"("Visible"=FALSE) -> ()  [unwired: 2 in, 2 out]
                    n615 = property on="Filename" class="Path"("Visible"=FALSE) -> ()  [unwired: 2 in, 2 out]
                    n616 = property on="Final" class="Digital (strict)"("Visible"=w354) -> ()  [unwired: 2 in, 2 out]
                    n617 = property on="Initial" class="Digital (strict)"("Visible"=w354) -> ()  [unwired: 2 in, 2 out]
                    n618 = property on="Scan Rate" class="Digital (strict)"("Visible"=w354) -> ()  [unwired: 2 in, 2 out]
                    n619 = property on="Acq. Frequency" class="Digital (strict)"("Visible"=w354) -> ()  [unwired: 2 in, 2 out]
                    n620 = property on="Cycles" class="DigNum (strict)"("Visible"=w354) -> ()  [unwired: 2 in, 2 out]
                    n621 = property on="Continuous" class="Boolean (strict)"("Visible"=w354) -> ()  [unwired: 2 in, 2 out]
                  }
                  frame #2 {
                    w359 = FALSE ("Visible")
                    (unwired) FALSE ("Visible")
                    w361 = TRUE ("Visible")
                    n622 = property on="Signal Frequency" class="Digital (strict)"("Visible"=w361) -> ()  [unwired: 2 in, 2 out]
                    n623 = property on="Amplitude" class="Digital (strict)"("Visible"=w361) -> ()  [unwired: 2 in, 2 out]
                    n624 = property on="DC Offset" class="Digital (strict)"("Visible"=w361) -> ()  [unwired: 2 in, 2 out]
                    n625 = property on="Acq. Frequency" class="Digital (strict)"("Visible"=w361) -> ()  [unwired: 2 in, 2 out]
                    n626 = property on="Cycles" class="DigNum (strict)"("Visible"=w361) -> ()  [unwired: 2 in, 2 out]
                    n627 = property on="Continuous" class="Boolean (strict)"("Visible"=w361) -> ()  [unwired: 2 in, 2 out]
                    n628 = property on="Duty Cycle" class="DigNum (strict)"("Visible"=TRUE) -> ()  [unwired: 2 in, 2 out]
                    n629 = property on="Phase Offset" class="Digital (strict)"("Visible"=FALSE) -> ()  [unwired: 2 in, 2 out]
                    n630 = property on="Filename" class="Path"("Visible"=FALSE) -> ()  [unwired: 2 in, 2 out]
                    n631 = property on="Final" class="Digital (strict)"("Visible"=w359) -> ()  [unwired: 2 in, 2 out]
                    n632 = property on="Initial" class="Digital (strict)"("Visible"=w359) -> ()  [unwired: 2 in, 2 out]
                    n633 = property on="Scan Rate" class="Digital (strict)"("Visible"=w359) -> ()  [unwired: 2 in, 2 out]
                  }
                  frame #3 {
                    w363 = TRUE ("Visible")
                    (unwired) FALSE ("Visible")
                    w364 = FALSE ("Visible")
                    # "Ramp"
                    n634 = property on="Signal Frequency" class="Digital (strict)"("Visible"=w364) -> ()  [unwired: 2 in, 2 out]
                    n635 = property on="Amplitude" class="Digital (strict)"("Visible"=w364) -> ()  [unwired: 2 in, 2 out]
                    n636 = property on="DC Offset" class="Digital (strict)"("Visible"=w364) -> ()  [unwired: 2 in, 2 out]
                    n637 = property on="Phase Offset" class="Digital (strict)"("Visible"=w364) -> ()  [unwired: 2 in, 2 out]
                    n638 = property on="Cycles" class="DigNum (strict)"("Visible"=w364) -> ()  [unwired: 2 in, 2 out]
                    n639 = property on="Continuous" class="Boolean (strict)"("Visible"=w364) -> ()  [unwired: 2 in, 2 out]
                    n640 = property on="Duty Cycle" class="DigNum (strict)"("Visible"=FALSE) -> ()  [unwired: 2 in, 2 out]
                    n641 = property on="Filename" class="Path"("Visible"=FALSE) -> ()  [unwired: 2 in, 2 out]
                    n642 = property on="Final" class="Digital (strict)"("Visible"=w363) -> ()  [unwired: 2 in, 2 out]
                    n643 = property on="Initial" class="Digital (strict)"("Visible"=w363) -> ()  [unwired: 2 in, 2 out]
                    n644 = property on="Scan Rate" class="Digital (strict)"("Visible"=w363) -> ()  [unwired: 2 in, 2 out]
                    n645 = property on="Acq. Frequency" class="Digital (strict)"("Visible"=w363) -> ()  [unwired: 2 in, 2 out]
                  }
                  frame #4 {
                    w368 = FALSE ("Visible")
                    w366 = TRUE ("Visible")
                    w370 = FALSE ("Visible")
                    # "Single Point"
                    n646 = property on="Signal Frequency" class="Digital (strict)"("Visible"=w370) -> ()  [unwired: 2 in, 2 out]
                    n647 = property on="Amplitude" class="Digital (strict)"("Visible"=w370) -> ()  [unwired: 2 in, 2 out]
                    n648 = property on="Phase Offset" class="Digital (strict)"("Visible"=w370) -> ()  [unwired: 2 in, 2 out]
                    n649 = property on="Cycles" class="DigNum (strict)"("Visible"=w370) -> ()  [unwired: 2 in, 2 out]
                    n650 = property on="Continuous" class="Boolean (strict)"("Visible"=w370) -> ()  [unwired: 2 in, 2 out]
                    n651 = property on="Acq. Frequency" class="Digital (strict)"("Visible"=w366) -> ()  [unwired: 2 in, 2 out]
                    n652 = property on="DC Offset" class="Digital (strict)"("Visible"=w366) -> ()  [unwired: 2 in, 2 out]
                    n653 = property on="Duty Cycle" class="DigNum (strict)"("Visible"=FALSE) -> ()  [unwired: 2 in, 2 out]
                    n654 = property on="Filename" class="Path"("Visible"=FALSE) -> ()  [unwired: 2 in, 2 out]
                    n655 = property on="Final" class="Digital (strict)"("Visible"=w368) -> ()  [unwired: 2 in, 2 out]
                    n656 = property on="Initial" class="Digital (strict)"("Visible"=w368) -> ()  [unwired: 2 in, 2 out]
                    n657 = property on="Scan Rate" class="Digital (strict)"("Visible"=w368) -> ()  [unwired: 2 in, 2 out]
                  }
                  frame #5 {
                    w372 = FALSE ("Visible")
                    w373 = TRUE ("Visible")
                    (unwired) FALSE ("Visible")
                    w374 = FALSE ("Visible")
                    # "From File"
                    n658 = property on="Signal Frequency" class="Digital (strict)"("Visible"=w374) -> ()  [unwired: 2 in, 2 out]
                    n659 = property on="Amplitude" class="Digital (strict)"("Visible"=w374) -> ()  [unwired: 2 in, 2 out]
                    n660 = property on="DC Offset" class="Digital (strict)"("Visible"=w374) -> ()  [unwired: 2 in, 2 out]
                    n661 = property on="Phase Offset" class="Digital (strict)"("Visible"=w374) -> ()  [unwired: 2 in, 2 out]
                    n662 = property on="Duty Cycle" class="DigNum (strict)"("Visible"=FALSE) -> ()  [unwired: 2 in, 2 out]
                    n663 = property on="Filename" class="Path"("Visible"=w373) -> ()  [unwired: 2 in, 2 out]
                    n664 = property on="Acq. Frequency" class="Digital (strict)"("Visible"=w373) -> ()  [unwired: 2 in, 2 out]
                    n665 = property on="Cycles" class="DigNum (strict)"("Visible"=w373) -> ()  [unwired: 2 in, 2 out]
                    n666 = property on="Continuous" class="Boolean (strict)"("Visible"=w373) -> ()  [unwired: 2 in, 2 out]
                    n667 = property on="Scan Rate" class="Digital (strict)"("Visible"=w372) -> ()  [unwired: 2 in, 2 out]
                    n668 = property on="Final" class="Digital (strict)"("Visible"=w372) -> ()  [unwired: 2 in, 2 out]
                    n669 = property on="Initial" class="Digital (strict)"("Visible"=w372) -> ()  [unwired: 2 in, 2 out]
                  }
                  frame #6 {
                  }
                }
              }
              frame #1 {
                n670 = case shown="True" w378 {
                  tunnel: w379 -> [_ w387]
                  tunnel: w377 -> [_ w382]
                  tunnel: w376 -> [_ w381]
                  tunnel: w375 -> [_ w380]
                  frame #0 {
                  }
                  frame #1 {
                    # "Nyquist Criterion"
                    n671 = local read "Signal Frequency"() -> (w383:dbl)
                    n672 = local read "Acq. Frequency"() -> (w384:dbl)
                    n673 = local read "Signal Type"() -> (w386:u16)
                    n674 = case shown="0, 1, 3, 4" w386 {
                      tunnel: w384 -> [_ w393]
                      tunnel: w383 -> [_ w391]
                      tunnel: [TRUE w389] -> w385
                      frame #0 {
                      }
                      frame #1 {
                        n675 = Multiply(x=2.0, y=w391) -> (x*y=w392:dbl)
                        n676 = Greater?(x=w393, y=w392) -> (0:w389:bool)
                      }
                    }
                    n677 = case shown="True" w385 {
                      tunnel: w383 -> [_ w417]
                      tunnel: w384 -> [_ w416]
                      tunnel: w387 -> [_ w413]
                      tunnel: w382 -> [_ w406]
                      tunnel: w381 -> [_ w405]
                      tunnel: w380 -> [_ w402]
                      frame #0 {
                        n678 = call "Nyquist Criterion"("Enable"=TRUE) -> ()  [unwired: 9 in, 2 out]
                      }
                      frame #1 {
                        w396 = 0 items=["SigTweakStyleReset", "SigTweakStyleContinue", "SigTweakStyleScale"] ("Tweak Style")
                        # "Check to see if the signal type changed,\nIf so, we want to RESET the tweak rather\nthan try and transition gracefully."
                        n679 = local read "Amplitude"() -> (w418:dbl)
                        n680 = local read "Continuous"() -> (w414:bool)
                        n681 = local read "Cycles"() -> (w415:u32)
                        n682 = local read "Phase Offset"() -> (w420:dbl)
                        n683 = local read "Duty Cycle"() -> (w425:dbl)
                        n684 = local read "DC Offset"() -> (w419:dbl)
                        n685 = local read "Scan Rate"() -> (w421:dbl)
                        n686 = local read "Final"() -> (w422:dbl)
                        n687 = local read "Initial"() -> (w423:dbl)
                        n688 = Not Equal?(x=w406, y=w405) -> (x != y?=w400:bool)
                        n689 = case shown="7" w413 {
                          selector: w413 -> [w437 w453 w480 w495 _ _ _]
                          tunnel: w414 -> [w439 w455 w482 _ _ w528 w544]
                          tunnel: w415 -> [w438 w454 w481 _ _ w527 w543]
                          tunnel: w416 -> [w436 w452 w479 w503 w519 w526 w549]
                          tunnel: w417 -> [w428 _ w470 _ _ _ _]
                          tunnel: w418 -> [w435 _ w478 _ _ _ _]
                          tunnel: w419 -> [w434 _ w477 _ w513 _ _]
                          tunnel: w420 -> [w433 _ w476 _ _ _ _]
                          tunnel: w421 -> [_ w451 _ w502 _ _ _]
                          tunnel: w422 -> [_ w450 _ w501 _ _ _]
                          tunnel: w423 -> [_ w449 _ w500 _ _ _]
                          tunnel: [w432 w447 w475 w497 w517 w523 dbl[] []] -> w411
                          tunnel: [w431 w448 w474 1 ("t") -1 ("t") w524 w542] -> w412
                          tunnel: [w430 w446 w473 w498 w516 w525 w548] -> w408
                          tunnel: [w429 w445 w472 w496 0 ("error") 0 ("error") 0 ("error")] -> w424
                          tunnel: w425 -> [_ _ w471 _ _ _ _]
                          tunnel: [w426 w442 w468 w485 w514 w521 w541] -> w397
                          tunnel: w402 -> [_ _ _ w486 _ _ _]
                          frame #0 {
                            w426 = 2 items=["SigTweakStyleReset", "SigTweakStyleContinue", "SigTweakStyleScale"] ("Tweak Style")
                            # "Sine, Cosine, Sawtooth"
                            n690 = Select(t=-1, s=w439, f=w438) -> (s? t:f=w431:u32)
                            n691 = Reciprocal(x=w428) -> (1/x=w427:dbl)
                            n692 = Reciprocal(x=w436) -> (1/x=w430:dbl)
                            n693 = Multiply(x=w436, y=w427) -> (x*y=w441:dbl)
                            n694 = call <vilib>:"Signal Generator by Duration.vi"("signal type"=w437, "duration"=w427, "# of samples"=w441, "frequency"=w428, "amplitude"=w435, "dc offset"=w434, "phase in"=w433) -> ("signal"=w432:dbl[], "error"=w429:i32)  [unwired: 5 in, 2 out]
                          }
                          frame #1 {
                            w442 = 0 items=["SigTweakStyleReset", "SigTweakStyleContinue", "SigTweakStyleScale"] ("Tweak Style")
                            # "Triangle"
                            n695 = Select(t=-1, s=w455, f=w454) -> (s? t:f=w448:u32)
                            n696 = Subtract(x=w450, y=w449) -> (x-y=w460:dbl)
                            n697 = Add(x=w450, y=w449) -> (x+y=w456:dbl)
                            n698 = Divide(x=w460, y=w451) -> (x/y=w465:dbl)
                            n699 = Divide(x=w460, y=2.0) -> (x/y=w459:dbl)
                            n700 = Divide(x=w456, y=2.0) -> (x/y=w458:dbl)
                            n701 = Reciprocal(x=w452) -> (1/x=w446:dbl)
                            n702 = Absolute Value(x=w465) -> (abs(x)=w464:dbl)
                            n703 = Multiply(x=w464, y=2.0) -> (x*y=w443:dbl)
                            n704 = Reciprocal(x=w443) -> (1/x=w444:dbl)
                            n705 = Multiply(x=w452, y=w443) -> (x*y=w467:dbl)
                            n706 = call <vilib>:"Signal Generator by Duration.vi"("signal type"=w453, "duration"=w443, "# of samples"=w467, "frequency"=w444, "amplitude"=w459, "dc offset"=w458, "phase in"=270.0) -> ("signal"=w447:dbl[], "error"=w445:i32)  [unwired: 5 in, 2 out]
                          }
                          frame #2 {
                            w468 = 2 items=["SigTweakStyleReset", "SigTweakStyleContinue", "SigTweakStyleScale"] ("Tweak Style")
                            # "Square Wave"
                            n707 = Select(t=-1, s=w482, f=w481) -> (s? t:f=w474:u32)
                            n708 = Reciprocal(x=w470) -> (1/x=w469:dbl)
                            n709 = Reciprocal(x=w479) -> (1/x=w473:dbl)
                            n710 = Multiply(x=w479, y=w469) -> (x*y=w484:dbl)
                            n711 = call <vilib>:"Signal Generator by Duration.vi"("signal type"=w480, "duration"=w469, "# of samples"=w484, "frequency"=w470, "amplitude"=w478, "dc offset"=w477, "phase in"=w476, "square wave duty cycle (%)"=w471) -> ("signal"=w475:dbl[], "error"=w472:i32)  [unwired: 4 in, 2 out]
                          }
                          frame #3 {
                            # "Ramp"
                            n712 = control-ref of="Initial"() -> (w490:refnum<vi>)
                            n713 = control-ref of="Scan Rate"() -> (w487:refnum<vi>)
                            n714 = Subtract(x=w501, y=w500) -> (x-y=w505:dbl)
                            n715 = Divide(x=w505, y=w502) -> (x/y=w504:dbl)
                            n716 = To More Generic Class(target class=w486, reference=w490) -> (generic class reference=w489:refnum<vi>)
                            n717 = To More Generic Class(target class=w486, reference=w487) -> (generic class reference=w488:refnum<vi>)
                            n718 = Absolute Value(x=w504) -> (abs(x)=w493:dbl)
                            n719 = Equal?(x=w486, y=w489) -> (x = y?=w491:bool)
                            n720 = Equal?(x=w486, y=w488) -> (x = y?=w492:bool)
                            n721 = Reciprocal(x=w503) -> (1/x=w498:dbl)
                            n722 = Reciprocal(x=w493) -> (1/x=w494:dbl)
                            n723 = case shown="False" w491 {
                              tunnel: w492 -> [w509 _]
                              tunnel: [w508 w512] -> w485
                              frame #0 {
                                n724 = case shown="False" w509 {
                                tunnel: [w510 w511] -> w508
                                frame #0 {
                                w510 = 1 items=["SigTweakStyleReset", "SigTweakStyleContinue", "SigTweakStyleScale"] ("Tweak Style")
                                }
                                frame #1 {
                                w511 = 2 items=["SigTweakStyleReset", "SigTweakStyleContinue", "SigTweakStyleScale"] ("Tweak Style")
                                }
                                }
                              }
                              frame #1 {
                                w512 = 0 items=["SigTweakStyleReset", "SigTweakStyleContinue", "SigTweakStyleScale"] ("Tweak Style")
                              }
                            }
                            n725 = Multiply(x=w503, y=w493) -> (x*y=w507:dbl)
                            n726 = call <vilib>:"Signal Generator by Duration.vi"("signal type"=w495, "duration"=w493, "# of samples"=w507, "frequency"=w494, "amplitude"=w505, "dc offset"=w500, "phase in"=0.0) -> ("signal"=w497:dbl[], "error"=w496:i32)  [unwired: 5 in, 2 out]
                          }
                          frame #4 {
                            w514 = 0 items=["SigTweakStyleReset", "SigTweakStyleContinue", "SigTweakStyleScale"] ("Tweak Style")
                            # "Single Point"
                            n727 = Reciprocal(x=w519) -> (1/x=w516:dbl)
                            n728 = Initialize Array(w513, 1 ("dimension size")) -> (w517:dbl[])
                          }
                          frame #5 {
                            w521 = 0 items=["SigTweakStyleReset", "SigTweakStyleContinue", "SigTweakStyleScale"] ("Tweak Style")
                            (unwired) TRUE ("convert eol (F)")
                            # "From File"
                            n729 = local read "Filename"() -> (w539:path)
                            n730 = call <vilib>:"Open_Create_Replace File.vi"("file path"=w539) -> ("error out"=w536:errorcluster, "file size (bytes)"=w537:i32, "new file path"=w538:path, "refnum"=w540:refnum<file>)  [unwired: 7 in]
                            n731 = local write "Filename"(w538) -> ()
                            n732 = Select(t=-1, s=w528, f=w527) -> (s? t:f=w524:u32)
                            n733 = Reciprocal(x=w526) -> (1/x=w525:dbl)
                            n734 = Read from Text File(file (use dialog)=w540, count=w537, error in=w536) -> (refnum out=w529:refnum<file>, text=w531:string, error out=w530:errorcluster)  [unwired: 1 in, 1 out]
                            n735 = local write "From File Refnum"(w529) -> ()
                            n736 = Close File(refnum=w529, error in=w530) -> ()  [unwired: 2 out]
                            n737 = local write "File Data"(w531) -> ()
                            n738 = Spreadsheet String To Array(delimiter (Tab)="\n", format string="%f", spreadsheet string=w531, array type (2D Dbl)=dbl[] [] ("initialized array")) -> (array=w523:dbl[])
                          }
                          frame #6 {
                            w541 = 0 items=["SigTweakStyleReset", "SigTweakStyleContinue", "SigTweakStyleScale"] ("Tweak Style")
                            n739 = Reciprocal(x=w549) -> (1/x=w548:dbl)
                            n740 = Select(t=-1, s=w544, f=w543) -> (s? t:f=w542:u32)
                          }
                        }
                        n741 = call <vilib>:"Error Cluster From Error Code.vi"("error code (0)"=w424) -> ("error out"=w395:errorcluster)  [unwired: 8 in]
                        n742 = control-ref of="Signal Type"() -> (w404:refnum<vi>)
                        n743 = To More Generic Class(target class=w402, reference=w404) -> (generic class reference=w403:refnum<vi>)
                        n744 = property on="Vs. T" class="WaveformChart (strict)"("X Scale.Offset and Multiplier:Multiplier"=w408) -> ()  [unwired: 2 in, 2 out]
                        n745 = Equal?(x=w402, y=w403) -> (x = y?=w399:bool)
                        n746 = And(x=w400, y=w399) -> (x .and. y?=w398:bool)
                        n747 = local read "Signal"() -> (w407:refnum<k7>)
                        n748 = Select(t=w396, s=w398, f=w397) -> (s? t:f=w401:i32)
                        n749 = call "SigArrayTweak.vi"("Signal IN"=w407, "Style"=w401, "Cycles"=w412, "Sample Rate"=w408, "Signal Array"=w411, "error in"=w395) -> ("error out"=w410:errorcluster)  [unwired: 8 in, 1 out]
                        n750 = Unbundle By Name(w410) -> ("status"=w409:bool)
                        n751 = call "Tweak Error"("Enable"=w409) -> ()  [unwired: 9 in, 2 out]
                      }
                    }
                  }
                }
              }
            }
          }
          event #5 {
            w561 = T13 0 items=["no dialog", "OK message", "continue or stop message", "OK message + warnings", "continue/stop + warnings"] ("type of dialog (OK msg:1)")
            n752 = event-data() -> ("CtlRef"=w551:refnum<vi>)  [unwired: 1 in, 5 out]
            n753 = property class="Bool (strict)"(reference=w551, "Value"=FALSE ("Device List Change")) -> ()  [unwired: 1 in, 2 out]
            n754 = local read "Device List"() -> (w560:refnum<k7>)
            n755 = local read "Section List"() -> (w558:string[])
            n756 = local read "Device"() -> (w559:u16)
            n757 = call "UpdateDeviceList.vi"("Section List"=w558, "Device"=w559, "Device List"=w560) -> ("error out"=w553:errorcluster, "New Section List"=w557:string[], "New Label List"=w555:string[], "New Device Index"=w554:i32)  [unwired: 5 in]
            n758 = local write "Index of Device (Device Change)"(w554) -> ()
            n759 = local write "Section List"(w557) -> ()
            n760 = Not Equal?(x=w554, y=-1) -> (x != y?=w564:bool)
            n761 = Select(t=w554, s=w564, f=0) -> (s? t:f=w565:i32)
            n762 = local read "Taking Data"() -> (w569:bool)
            n763 = Not(x=w564) -> (.not. x?=w563:bool)
            n764 = property on="Device" class="Ring (strict)"(error in=w553, "Strings []"=w555, "Value (Signaling)"=w565) -> (error out=w556:errorcluster)  [unwired: 1 in, 1 out]
            n765 = And(x=w563, y=w569) -> (x .and. y?=w568:bool)
            n766 = case shown="True" w568 {
              tunnel: w556 -> [w580 w582]
              tunnel: [w580 w582] -> w562
              frame #0 {
              }
              frame #1 {
                # "Stop and notify User"
                n767 = local write "Start/Stop"(FALSE ("Start/Stop")) -> ()
                n768 = local write "Device Open"(FALSE ("Device Gone")) -> ()
                n769 = local write "Device Gone"(TRUE ("Device Gone")) -> ()
              }
            }
            n770 = local read "[user-defined descriptions]"() -> (w571:string[])
            n771 = local read "[user-defined codes]"() -> (w570:u32[])
            n772 = local read "Taking Data"() -> (w552:bool)
            n773 = call <vilib>:"General Error Handler.vi"("[user-defined codes]"=w570, "[user-defined descriptions]"=w571, "type of dialog (OK msg:1)"=w561, "error in (no error)"=w562) -> ("error out"=w572:errorcluster)  [unwired: 7 in, 4 out]
            n774 = case shown="False" w552 {
              tunnel: w572 -> [w573 w577]
              frame #0 {
                n775 = case shown="No Error" w573 {
                  frame #0 {
                    w574 = u8 0 ("Disabled")
                    # "Enable appropriate menu stuff"
                    n776 = property on="Start/Stop" class="Bool (strict)"("Disabled"=w574) -> ()  [unwired: 2 in, 2 out]
                    n777 = property on="Signal Type" class="Ring (strict)"("Disabled"=w574) -> ()  [unwired: 2 in, 2 out]
                    n778 = property on="Device" class="Ring (strict)"("Disabled"=w574) -> ()  [unwired: 2 in, 2 out]
                    n779 = property on="CtrlMode" class="Ring (strict)"("Disabled"=w574) -> ()  [unwired: 2 in, 2 out]
                    n780 = property on="I/E Range" class="Ring (strict)"("Disabled"=w574) -> ()  [unwired: 2 in, 2 out]
                    n781 = property on="Vch Range" class="Ring (strict)"("Disabled"=w574) -> ()  [unwired: 2 in, 2 out]
                    n782 = property on="Ich Range" class="Ring (strict)"("Disabled"=w574) -> ()  [unwired: 2 in, 2 out]
                    n783 = property on="Vch Filter" class="Ring (strict)"("Disabled"=w574) -> ()  [unwired: 2 in, 2 out]
                    n784 = property on="Ich Filter" class="Ring (strict)"("Disabled"=w574) -> ()  [unwired: 2 in, 2 out]
                    n785 = property on="Vch Offset" class="DigNum (strict)"("Disabled"=w574) -> ()  [unwired: 2 in, 2 out]
                    n786 = property on="Ich Offset" class="DigNum (strict)"("Disabled"=w574) -> ()  [unwired: 2 in, 2 out]
                    n787 = property on="I/E Stability" class="Ring (strict)"("Disabled"=w574) -> ()  [unwired: 2 in, 2 out]
                    n788 = property on="CA Speed" class="Ring (strict)"("Disabled"=w574) -> ()  [unwired: 2 in, 2 out]
                  }
                  frame #1 {
                    w576 = u16 0 items=[""] ("Device")
                    w575 = u8 2 ("Disabled")
                    # "Disable appropriate menu stuff"
                    n789 = property on="Start/Stop" class="Bool (strict)"("Disabled"=w575) -> ()  [unwired: 2 in, 2 out]
                    n790 = property on="CtrlMode" class="Ring (strict)"("Disabled"=w575) -> ()  [unwired: 2 in, 2 out]
                    n791 = property on="Device" class="Ring (strict)"("Disabled"=w575, "Value"=w576) -> ()  [unwired: 2 in, 2 out]
                    n792 = property on="I/E Range" class="Ring (strict)"("Disabled"=w575, "Value"=w576) -> ()  [unwired: 2 in, 2 out]
                    n793 = property on="Vch Range" class="Ring (strict)"("Disabled"=w575, "Value"=w576) -> ()  [unwired: 2 in, 2 out]
                    n794 = property on="Ich Range" class="Ring (strict)"("Disabled"=w575, "Value"=w576) -> ()  [unwired: 2 in, 2 out]
                    n795 = property on="Vch Filter" class="Ring (strict)"("Disabled"=w575, "Value"=w576) -> ()  [unwired: 2 in, 2 out]
                    n796 = property on="Ich Filter" class="Ring (strict)"("Disabled"=w575, "Value"=w576) -> ()  [unwired: 2 in, 2 out]
                    n797 = property on="Vch Offset" class="DigNum (strict)"("Disabled"=w575) -> ()  [unwired: 2 in, 2 out]
                    n798 = property on="Ich Offset" class="DigNum (strict)"("Disabled"=w575) -> ()  [unwired: 2 in, 2 out]
                    n799 = property on="I/E Stability" class="Ring (strict)"("Disabled"=w575) -> ()  [unwired: 2 in, 2 out]
                    n800 = property on="CA Speed" class="Ring (strict)"("Disabled"=w575) -> ()  [unwired: 2 in, 2 out]
                  }
                }
              }
              frame #1 {
                n801 = case shown="No Error" w577 {
                  frame #0 {
                  }
                  frame #1 {
                    w579 = u16 0 items=[""] ("Device")
                    w578 = u8 2 ("Disabled")
                    # "Disable appropriate menu stuff"
                    n802 = property on="Start/Stop" class="Bool (strict)"("Disabled"=w578) -> ()  [unwired: 2 in, 2 out]
                    n803 = property on="CtrlMode" class="Ring (strict)"("Disabled"=w578) -> ()  [unwired: 2 in, 2 out]
                    n804 = property on="Device" class="Ring (strict)"("Disabled"=w578, "Value"=w579) -> ()  [unwired: 2 in, 2 out]
                    n805 = property on="I/E Range" class="Ring (strict)"("Disabled"=w578, "Value"=w579) -> ()  [unwired: 2 in, 2 out]
                    n806 = property on="Vch Range" class="Ring (strict)"("Disabled"=w578, "Value"=w579) -> ()  [unwired: 2 in, 2 out]
                    n807 = property on="Ich Range" class="Ring (strict)"("Disabled"=w578, "Value"=w579) -> ()  [unwired: 2 in, 2 out]
                    n808 = property on="Vch Filter" class="Ring (strict)"("Disabled"=w578, "Value"=w579) -> ()  [unwired: 2 in, 2 out]
                    n809 = property on="Ich Filter" class="Ring (strict)"("Disabled"=w578, "Value"=w579) -> ()  [unwired: 2 in, 2 out]
                    n810 = property on="Vch Offset" class="DigNum (strict)"("Disabled"=w578) -> ()  [unwired: 2 in, 2 out]
                    n811 = property on="Ich Offset" class="DigNum (strict)"("Disabled"=w578) -> ()  [unwired: 2 in, 2 out]
                    n812 = property on="I/E Stability" class="Ring (strict)"("Disabled"=w578) -> ()  [unwired: 2 in, 2 out]
                    n813 = property on="CA Speed" class="Ring (strict)"("Disabled"=w578) -> ()  [unwired: 2 in, 2 out]
                  }
                }
              }
            }
          }
          event #6 {
            n814 = event-data() -> ("NewVal"=w586:u16)  [unwired: 1 in, 5 out]
            n815 = local read "Section List"() -> (w587:string[])
            n816 = Index Array(array=w587, index=w586) -> (element=w585:string)
            n817 = property on="Section" class="Str"("Value (Signaling)"=w585) -> ()  [unwired: 2 in, 2 out]
          }
          event #7 {
            n818 = event-data() -> ("OldVal"=w589:string, "NewVal"=w588:string)  [unwired: 1 in, 4 out]
            n819 = Not Equal?(x=w589, y=w588) -> (x != y?=w590:bool)
            n820 = case shown="True" w590 {
              tunnel: w588 -> [_ w597]
              frame #0 {
              }
              frame #1 {
                n821 = local read "Device Open"() -> (w602:bool)
                n822 = local read "Pstat"() -> (w604:refnum<k7>)
                n823 = case shown="True" w602 {
                  tunnel: w604 -> [w649 w653]
                  tunnel: [w649 w652] -> w603
                  tunnel: [errorcluster {"status"=FALSE, "code"=0, "source"=""} ("error out") w650] -> w601
                  frame #0 {
                  }
                  frame #1 {
                    n824 = invoke class="IGamryPstat" method="Close"(reference=w653, "Safe"=TRUE) -> (reference out=w652:refnum<k7>, error out=w650:errorcluster)  [unwired: 2 in, 2 out]
                  }
                }
                n825 = invoke class="IGamryPstat" method="Init"(reference=w603, error in=w601, "Section"=w597) -> (reference out=w600:refnum<k7>, error out=w599:errorcluster)  [unwired: 1 in, 2 out]
                n826 = invoke class="IGamryPstat" method="Open"(reference=w600, error in=w599) -> (reference out=w593:refnum<k7>, error out=w598:errorcluster)  [unwired: 1 in, 1 out]
                n827 = case shown="No Error" w598 {
                  selector: w598 -> [w644 w646]
                  tunnel: [w644 w646] -> w594
                  frame #0 {
                    n828 = local write "Device Open"(TRUE ("Device Open")) -> ()
                  }
                  frame #1 {
                    n829 = local write "Device Open"(FALSE ("Device Open")) -> ()
                  }
                }
                n830 = call "HardwareRangeStrings.vi"("error in (no error)"=w594, "Pstat IN"=w593) -> ("error out"=w595:errorcluster, "Hardware Strings"=w591:T7, "Pstat OUT"=w592:refnum<k7>)  [unwired: 7 in]
                n831 = Unbundle By Name(w591) -> ("I/E Ranges"=w636:string[], "First I/E Range"=w624:i32, "VchRanges"=w638:string[], "IchRanges"=w637:string[], "VchFilters"=w635:string[], "IchFilters"=w634:string[], "Family"=w596:string, "CA Speeds"=w627:string[])  [unwired: 2 out]
                n832 = invoke class="IGamryPstat" method="CtrlMode"(reference=w592, error in=w595) -> (reference out=w630:refnum<k7>, error out=w631:errorcluster, "CtrlMode"=w639:i32)  [unwired: 1 in]
                n833 = local write "CtrlMode"(w639) -> ()
                n834 = invoke class="IGamryPstat" method="IchRange"(reference=w630, error in=w631) -> (reference out=w628:refnum<k7>, error out=w629:errorcluster, "IchRange"=w641:i32)  [unwired: 1 in]
                n835 = property on="I/E Range" class="Ring (strict)"("Strings []"=w636) -> ()  [unwired: 2 in, 2 out]
                n836 = property on="Vch Range" class="Ring (strict)"("Strings []"=w638) -> ()  [unwired: 2 in, 2 out]
                n837 = property on="Ich Range" class="Ring (strict)"("Strings []"=w637) -> ()  [unwired: 2 in, 2 out]
                n838 = property on="Vch Filter" class="Ring (strict)"("Strings []"=w635) -> ()  [unwired: 2 in, 2 out]
                n839 = property on="Ich Filter" class="Ring (strict)"("Strings []"=w634) -> ()  [unwired: 2 in, 2 out]
                n840 = property on="CA Speed" class="Ring (strict)"("Strings []"=w627) -> ()  [unwired: 2 in, 2 out]
                n841 = local write "Family"(w596) -> ()
                n842 = local write "Ich Range"(w641) -> ()
                n843 = invoke class="IGamryPstat" method="VchRange"(reference=w628, error in=w629) -> (reference out=w611:refnum<k7>, error out=w612:errorcluster, "VchRange"=w640:i32)  [unwired: 1 in]
                n844 = invoke class="IGamryPstat" method="IchFilter"(reference=w611, error in=w612) -> (reference out=w617:refnum<k7>, error out=w618:errorcluster, "IchFilter"=w616:i32)  [unwired: 1 in]
                n845 = local write "Ich Filter"(w616) -> ()
                n846 = invoke class="IGamryPstat" method="VchFilter"(reference=w617, error in=w618) -> (reference out=w609:refnum<k7>, error out=w610:errorcluster, "VchFilter"=w615:i32)  [unwired: 1 in]
                n847 = invoke class="IGamryPstat" method="IchOffset"(reference=w609, error in=w610) -> (reference out=w620:refnum<k7>, error out=w619:errorcluster, "IchOffset"=w614:sgl)  [unwired: 1 in]
                n848 = local write "Ich Offset"(w614) -> ()
                n849 = invoke class="IGamryPstat" method="VchOffset"(reference=w620, error in=w619) -> (reference out=w607:refnum<k7>, error out=w608:errorcluster, "VchOffset"=w613:sgl)  [unwired: 1 in]
                n850 = invoke class="IGamryPstat" method="CASpeed"(reference=w607, error in=w608) -> (reference out=w626:refnum<k7>, error out=w625:errorcluster, "CASpeed"=w622:i32)  [unwired: 1 in]
                n851 = local write "CA Speed"(w622) -> ()
                n852 = invoke class="IGamryPstat" method="IEStability"(reference=w626, error in=w625) -> (reference out=w605:refnum<k7>, error out=w606:errorcluster, "IEStability"=w623:i32)  [unwired: 1 in]
                n853 = local write "I/E Stability"(w623) -> ()
                n854 = local write "Vch Range"(w640) -> ()
                n855 = local write "Vch Filter"(w615) -> ()
                n856 = local write "Vch Offset"(w613) -> ()
                n857 = invoke class="IGamryPstat" method="IERange"(reference=w605, error in=w606) -> (error out=w621:errorcluster, "IERange"=w642:i32)  [unwired: 1 in, 1 out]
                n858 = local read "[user-defined descriptions]"() -> (w632:string[])
                n859 = local read "[user-defined codes]"() -> (w633:u32[])
                n860 = Subtract(x=w642, y=w624) -> (x-y=w643:i32)
                n861 = local write "I/E Range"(w643) -> ()
                n862 = local write "First I/E Range"(w624) -> ()
                n863 = call <vilib>:"General Error Handler.vi"("[user-defined codes]"=w633, "[user-defined descriptions]"=w632, "error in (no error)"=w621) -> ()  [unwired: 8 in, 5 out]
              }
            }
          }
        }
        n864 = local read "Close"() -> (w165:bool)
        n865 = Not(x=w165) -> (.not. x?=w164:bool)
      }
    }
    frame #3 {
      w1077 = 0.0
      w1074 = u8 0 ("Disabled")
      w1075 = u16 0 items=[""] ("I/E Range")
      w1082 = 0 ("First I/E Range")
      w1076 = string[] [] ("Strings []")
      w1080 = FALSE ("Begin")
      # "Reset Buttons and Variables"
      n866 = local write "Cell State"(w1080) -> ()
      n867 = local write "Vch Autorange"(w1080) -> ()
      n868 = local write "Ich Autorange"(w1080) -> ()
      n869 = local write "VchOffsetEnable"(w1080) -> ()
      n870 = local write "Device List Change"(w1080) -> ()
      n871 = local write "I/E Autorange"(w1080) -> ()
      n872 = local write "IchOffsetEnable"(w1080) -> ()
      n873 = local write "Start/Stop"(w1080) -> ()
      n874 = local write "Close"(w1080) -> ()
      n875 = local write "Section"("" ("Section")) -> ()
      n876 = property on="Ich Offset" class="DigNum (strict)"("Value"=w1077, "Disabled"=w1074) -> ()  [unwired: 2 in, 2 out]
      n877 = property on="Device" class="Ring (strict)"("Strings []"=w1076, "Value"=w1075, "Disabled"=w1074) -> ()  [unwired: 2 in, 2 out]
      n878 = property on="CtrlMode" class="Ring (strict)"("Value"=w1075, "Disabled"=w1074) -> ()  [unwired: 2 in, 2 out]
      n879 = property on="Vch Offset" class="DigNum (strict)"("Value"=w1077, "Disabled"=w1074) -> ()  [unwired: 2 in, 2 out]
      n880 = property on="I/E Range" class="Ring (strict)"("Strings []"=w1076, "Value"=w1075, "Disabled"=w1074) -> ()  [unwired: 2 in, 2 out]
      n881 = property on="CA Speed" class="Ring (strict)"("Strings []"=w1076, "Value"=w1075, "Disabled"=w1074) -> ()  [unwired: 2 in, 2 out]
      n882 = property on="Ich Filter" class="Ring (strict)"("Strings []"=w1076, "Value"=w1075, "Disabled"=w1074) -> ()  [unwired: 2 in, 2 out]
      n883 = property on="I/E Range" class="Ring (strict)"("Strings []"=w1076, "Value"=w1075, "Disabled"=w1074) -> ()  [unwired: 2 in, 2 out]
      n884 = property on="Vch Range" class="Ring (strict)"("Strings []"=w1076, "Value"=w1075, "Disabled"=w1074) -> ()  [unwired: 2 in, 2 out]
      n885 = property on="Ich Range" class="Ring (strict)"("Strings []"=w1076, "Value"=w1075, "Disabled"=w1074) -> ()  [unwired: 2 in, 2 out]
      n886 = property on="Vch Filter" class="Ring (strict)"("Strings []"=w1076, "Value"=w1075, "Disabled"=w1074) -> ()  [unwired: 2 in, 2 out]
      n887 = property on="I/E Autorange" class="Boolean (strict)"("Disabled"=w1074) -> ()  [unwired: 2 in, 2 out]
      n888 = local write "First I/E Range"(w1082) -> ()
      n889 = local write "Device"(w1082) -> ()
      n890 = local read "Device List Change Callback"() -> (w1079:refnum<k27>)
      n891 = Not A Number/Path/Refnum?(number/path/refnum=w1079) -> (NaN/Path/Refnum?=w1078:bool)
      n892 = case shown="False" w1078 {
        tunnel: w1079 -> [w1083 _]
        frame #0 {
          n893 = Unregister For Events(event registration refnum=w1083) -> ()  [unwired: 1 in, 1 out]
        }
        frame #1 {
        }
      }
    }
  }
  n894 = while {
    stop <- w1087 continue-if-true
    n895 = local read "milliseconds to wait"() -> (w1084:u32)
    n896 = Current VI's Menubar() -> (w1085:refnum<k9>)
    n897 = local read "Close"() -> (w1088:bool)
    n898 = Get Menu Selection(0:w1085) -> (6:w1086:string)  [unwired: 3 in, 4 out]
    n899 = Wait (ms)(milliseconds to wait=w1084) -> ()  [unwired: 1 out]
    n900 = Not(x=w1088) -> (.not. x?=w1087:bool)
    n901 = case shown="\"MENU_About_VFP\"" w1086 {
      frame #0 {
      }
      frame #1 {
        n902 = local read "Version"() -> (w1089:string)
        n903 = Concatenate Strings("Virtual Front Panel\nVersion " ("message"), w1089, "\nCopyright 2010\nGamry Instruments, Inc." ("message")) -> (w1092:string)
        n904 = One Button Dialog(message=w1092) -> ()  [unwired: 1 in, 1 out]
      }
      frame #2 {
        w1093 = T13 1 items=["no dialog", "OK message", "continue or stop message", "OK message + warnings", "continue/stop + warnings"] ("type of dialog (OK msg:1)")
        n905 = property class="App"() -> ("Application:Kind"=w1095:T12, "Application:Directory Path"=w1094:path)  [unwired: 2 in, 2 out]
        n906 = case shown="\"Development System\"" w1095 {
          tunnel: [w1100 w1102] -> w1099
          tunnel: w1094 -> [_ w1102]
          frame #0 {
            n907 = Current VI's Path() -> (path=w1101:path)
            n908 = Strip Path(path=w1101) -> (stripped path=w1100:path)  [unwired: 1 out]
          }
          frame #1 {
          }
        }
        n909 = Build Path(base path=w1099, name or relative path="VFP600 Manual.pdf") -> (appended path=w1097:path)
        n910 = call <vilib>:"Open Acrobat Document.vi"("acrobat document"=w1097) -> ("error out"=w1096:errorcluster)  [unwired: 6 in]
        n911 = call <vilib>:"Simple Error Handler.vi"("type of dialog (OK msg:1)"=w1093, "error in (no error)"=w1096) -> ()  [unwired: 3 in, 5 out]
      }
    }
    n912 = event shown="[1] Panel Close?" {
      selector: _ -> [_ _ _]
      dyn-events: _ -> [_ _ _]
      timeout: w1084 -> [_ _ _]
      event #0 {
        # "This event is duplicated in Panel Close?"
        n913 = event-data() -> ()  [unwired: 1 in, 5 out]
        n914 = local read "Confirm Exit?"() -> (w1105:bool)
        n915 = local read "Taking Data"() -> (w1104:bool)
        n916 = Or(x=w1105, y=w1104) -> (x .or. y?=w1103:bool)
        n917 = case shown="True" w1103 {
          tunnel: [TRUE ("T button?") w1109] -> w1107
          frame #0 {
          }
          frame #1 {
            n918 = Two Button Dialog(message="Are you sure you would like to quit?", 1:"No" ("F button name (\"Cancel\")"), 2:"Yes" ("T button name (\"OK\")")) -> (T button?=w1109:bool)
          }
        }
        n919 = case shown="True" w1107 {
          frame #0 {
          }
          frame #1 {
            n920 = property class="App"() -> ("Application:Kind"=w1113:T12)  [unwired: 2 in, 2 out]
            n921 = case shown="\"Development System\"" w1113 {
              frame #0 {
                n922 = local write "Start/Stop"(FALSE) -> ()
                n923 = local write "Close"(TRUE) -> ()
              }
              frame #1 {
                n924 = Quit LabVIEW(quit? (T)=TRUE) -> ()
              }
            }
          }
        }
        n925 = event-data("Discard?"=TRUE) -> ()  [unwired: 2 in, 1 out]
      }
      event #1 {
        # "This event is duplicated in Application Exit?"
        n926 = event-data() -> ()  [unwired: 1 in, 4 out]
        n927 = local read "Confirm Exit?"() -> (w1119:bool)
        n928 = local read "Taking Data"() -> (w1118:bool)
        n929 = Or(x=w1119, y=w1118) -> (x .or. y?=w1117:bool)
        n930 = case shown="True" w1117 {
          tunnel: [TRUE ("T button?") w1123] -> w1121
          frame #0 {
          }
          frame #1 {
            n931 = Two Button Dialog(message="Are you sure you would like to quit?", 1:"No" ("F button name (\"Cancel\")"), 2:"Yes" ("T button name (\"OK\")")) -> (T button?=w1123:bool)
          }
        }
        n932 = case shown="True" w1121 {
          frame #0 {
          }
          frame #1 {
            n933 = property class="App"() -> ("Application:Kind"=w1127:T12)  [unwired: 2 in, 2 out]
            n934 = case shown="\"Development System\"" w1127 {
              frame #0 {
                n935 = local write "Start/Stop"(FALSE) -> ()
                n936 = local write "Close"(TRUE) -> ()
              }
              frame #1 {
                n937 = Quit LabVIEW(quit? (T)=TRUE) -> ()
              }
            }
          }
        }
        n938 = event-data("Discard?"=TRUE) -> ()  [unwired: 1 in, 1 out]
      }
      event #2 {
        n939 = event-data() -> ()  [unwired: 1 in, 3 out]
      }
    }
  }
  "Confirm Exit?" <- FALSE
  "Version" <- "5.62" ("Version")
  "Voltage Overload" <- w1
  "Current Overload" <- w1
  "Control Amp Overload" <- w1
